vi "Steuerprogramm-Fr-13-01-17.vi"() -> ()   [LabVIEW 2010]
uses:
  Emil/Licor-Steuerung/HAGAR V/Licor-Steuerung/display/GUI_Cluster_sdv.ctl
  Emil/Licor-Steuerung/HAGAR V/Licor-Steuerung/display/GUI_Cluster_Parameter.ctl
  Emil/Licor-Steuerung/HAGAR V/Licor-Steuerung/control/Licor-Commands.ctl
  Emil/Licor-Steuerung/HAGAR V/Licor-Steuerung/control/Licor-Parameter.ctl
  Emil/Licor-Steuerung/LicorLI7000/conventions/Licor-Source.ctl
  Emil/Licor-Steuerung/HAGAR V/Licor-Steuerung/control/Licor-Pump.ctl
  Emil/Licor-Steuerung/HAGAR V/Licor-Steuerung/display/GUI_Cluster_Graph.ctl
  Emil/Licor-Steuerung/HAGAR V/Licor-Steuerung/control/Licor-Sequences.ctl
  <vilib>/rvi/interface/nirviMethod/nirviMethod.xnode
  C:/Users/HAGAR-IV/Desktop/Zeugs/markus/version feb 2012/FPGA Bitfiles/pertrasgcfpga2_FPGATarget_FPGA-Programm-01_A75D3647.lvbitx
  C:/Users/HAGAR-IV/Desktop/Zeugs/Johnny/pertrasgc fpga/FPGA-Programm-01-17.vi
  <vilib>/rvi/interface/common/niFpgaNodeNameForErrorReporting.ctl
  <vilib>/rvi/errors/niLvFpgaWhatHappensToTopLevelVI.ctl
  <vilib>/rvi/interface/nirviReadWriteControl/nirviReadWriteControl.xnode
  <vilib>/rvi/interface/nirviCloseFPGA/nirviCloseFPGA.xnode
  GVProbenvol.vi
  GVZeitenZyklen.vi
  GVECDs.vi
  GVZwangs.vi
  GVMethodenwechsel.vi
  GVTrapsMachs.vi
  GVHK1Hz.vi
  GVAIs.vi
  gvbooleschRT.vi
  GVMetavariablen.vi
  GVVentilposition.vi
  GVHorstSP.vi
  GVMWHorst.vi
  GVHeizenLH.vi
  <vilib>/Utility/error.llb/Error Cluster From Error Code.vi
  <vilib>/rvi/errors/niLvFpgaAdjustHostInterfaceError.vi
  GVaktuelleTDMS.vi
  Emil/Licor-Steuerung/HAGAR V/Licor-Steuerung/control/Emulate Licor output GV.vi
  GVChroms.vi
  GVZwangsMPV.vi
  <vilib>/FPGAPlugInAG/cRIO-9114/niLvFpga_Close_cRIO-9114.vi
  NiFpgaLv.dll
  Emil/Licor-Steuerung/HAGAR V/Licor-Steuerung/Licor-Steuerung.lvlib
  Emil/Licor-Steuerung/LicorLI7000/LicorLI7000.lvlib
panel:
  in  "Methode speichern":bool
  out "ZyklusNummernGesamt":i32[](array[numeric])
  in  "veränderte Methode benutzen":bool
  in  "Methode verändern":bool
  out "ZyklusNummern":i32[](array[numeric])
  out "Big Ben, Methodenzeit, Zykluszeit0, Zykluszeit1, Zykluszeit2A, Zykluszeit2B":i32[](array[numeric])
  in  "global stop RT":bool
  in  "Methode":i32(ring) items=["Bedingsmethode", "Startmethode", "Meßmodus", "Shut-up-Methode", "Test", "HAG2 1/2", "Startmethode", "HAG2 1/2 Aufwärmen", "LicorDruckProfil1", "LicorDruckProfil2", "LicorDruckProfil0", "LicorDruckProfil3"]
  in  "Registerkarte":T1(tab)
  out "SHOK?":bool[](array[boolean])
  out "schnelle Heizungen":string[](array[string])
  out "schnelle Heizungen":dbl[](array[numeric])
  out "HorstOK?":bool[](array[boolean])
  out "AIs3OK?":bool[](array[boolean])
  out "AIs1OK?":bool[](array[boolean])
  out "AIs1":dbl[](array[numeric])
  out "AIs1":string[](array[string])
  out "AIs2":string[](array[string])
  out "AIs3":string[](array[string])
  out "AIs2":dbl[](array[numeric])
  out "AIs3":dbl[](array[numeric])
  out "Metavariablen":string[](array[string])
  out "Metavariablen":dbl[](array[numeric])
  out "MWHorst":dbl[](array[numeric])
  out "HorstRegler":string[](array[string])
  out "AIs2OK?":bool[](array[boolean])
  out "Ventilposition":i32=1 min=1 max=6 step=1
  out "MVOK?":bool[](array[boolean])
  out "Housekeeping1":cluster{dbl[], dbl[]}(graph)
  in  "Zeitachse1":i32(ring)=1 items=["Zykluszeit [s] Mod0", "Zykluszeit [s] Mod1", "Zykluszeit [s] Mod2A", "Zykluszeit [s] Mod2B"]
  in  "dargestellte Größe 1":i32(ring)=1 items=["T1-Trap1 [°C]", "T1-Trap2 [°C]", "T1-StirlingKühlkopf [°C]", "T1-PreCol1 [°C]", "T1-PreCol2 [°C]", "T1-MainCol1a [°C]", "T1-MainCol1b [°C]", "T1-MainCol2a [°C]", "T1-MainCol2b [°C]", "T1-Bronkhorst1a [°C]", "T1-Bronkhorst1b [°C]", "T1-Bronkhorst2a [°C]", "T1-Bronkhorst2b [°C]", "T1-2Pos1B [°C]", "T1-Spare9", "T1-2Pos1A [°C]", "T1-Spare10", "T1-TurboPump [°C]", "T1-StirlingPlatine [°C]", "T1-Spare5", "T1-Spare6", "T1-Spare7", "T1-Spare8", "F1-MFM1", "F1-MFM0D [mL]", "P1-HeliumHP [bara]", "P1-HeliumLP [bara]", "P1-PumpVordruck [mbara]", "TurboSpeed", "I1-MS-AC [A]", "I1-Trap1 [A]", "I1-Trap2 [A]", "T2-ECD1a", "T2-ECD1b", "T2-ECD2a", "T2-ECD2b", "T2-Col1a", "T2-Col1b", "T2-Col2a", "T2-Col2b", "T2-Spare1", "T2-Spare2", "T2-Oven_a", "T2-Oven_b", "T2-Spare3", "T2-Spare4", "T2-Spare5", "F2-MFM0", "F2-MFM2A", "F2-MFM2B", "P2-N2O_HP", "P2-N2O_LP", "P2-CO2_HP", "P2-CO2_LP", "AI-Spare1", "FL-MFM1000mL", "AI-Spare3", "AI-Spare4", "StirlingAlarm", "StirlingEmerg.", "AI-Spare7", "AI-Spare8", "AI-Spare9", "FL-MFM30mL", "T0-DC/DC5", "I0-24V_M0", "I0-48V_M1", "I0-24V_M1", "I0-28V_M2", "T0-Spare3", "T0-Spare2", "T0-Spare4", "T0-DC/DC7", "I0-20V_Laptop", "I0-28V_M1", "I0-24V_M2", "I0-12V_Licor", "T0-Spare1", "T0-Drier", "T0-Spare5", "F0-MFM0A [L]", "TL-Licor_a", "P0-Span-HP", "P0-spare1", "P0-Stickstoff-LP", "P0-Helium-LP", "P0-Cal-HP", "P0-P9Tavco[bar]", "F0-MFM0B [L]", "TL-Licor_b", "P0-Span-LP", "P0-spare2", "P0-Stickstoff-HP", "P0-Helium-HP", "P0-Cal-LP", "F0-MFM3", "TemperaturTrap1[°C]", "TemperaturTrap2[°C]", "TemperaturPreMach1[°C]", "TemperaturPreMach2[°C]", "TemperaturMainMach1[°C]", "TemperaturMainMach2[°C]", "PrC0 [bara]", "PrC0-Licor [bara]", "PrC1-Säule1 [bara]", "PrC1-Säule2 [bara]", "MFC1-Sample [ml/min]", "PrC1-BackFlush1 [bara]", "PrC1-BackFlush2 [bara]", "MFC1-Reaktant [l/min]", "MFC2A[ml/min]", "MFC2B[ml/min]", "MFC2C[ul/min]", "PrC2A[bara]", "MFC2D[ml/min]", "MFC2E[ml/min]", "PrC2B[bara]"]
  out "Housekeeping2":cluster{dbl[], dbl[]}(graph)
  in  "Zeitachse2":i32(ring)=1 items=["Zykluszeit [s] Mod0", "Zykluszeit [s] Mod1", "Zykluszeit [s] Mod2A", "Zykluszeit [s] Mod2B"]
  in  "dargestellte Größe 2":i32(ring)=1 items=["T1-Trap1 [°C]", "T1-Trap2 [°C]", "T1-StirlingKühlkopf [°C]", "T1-PreCol1 [°C]", "T1-PreCol2 [°C]", "T1-MainCol1a [°C]", "T1-MainCol1b [°C]", "T1-MainCol2a [°C]", "T1-MainCol2b [°C]", "T1-Bronkhorst1a [°C]", "T1-Bronkhorst1b [°C]", "T1-Bronkhorst2a [°C]", "T1-Bronkhorst2b [°C]", "T1-2Pos1B [°C]", "T1-Spare9", "T1-2Pos1A [°C]", "T1-Spare10", "T1-TurboPump [°C]", "T1-StirlingPlatine [°C]", "T1-Spare5", "T1-Spare6", "T1-Spare7", "T1-Spare8", "F1-MFM1", "F1-MFM0D [mL]", "P1-HeliumHP [bara]", "P1-HeliumLP [bara]", "P1-PumpVordruck [mbara]", "TurboSpeed", "I1-MS-AC [A]", "I1-Trap1 [A]", "I1-Trap2 [A]", "T2-ECD1a", "T2-ECD1b", "T2-ECD2a", "T2-ECD2b", "T2-Col1a", "T2-Col1b", "T2-Col2a", "T2-Col2b", "T2-Spare1", "T2-Spare2", "T2-Oven_a", "T2-Oven_b", "T2-Spare3", "T2-Spare4", "T2-Spare5", "F2-MFM0", "F2-MFM2A", "F2-MFM2B", "P2-N2O_HP", "P2-N2O_LP", "P2-CO2_HP", "P2-CO2_LP", "AI-Spare1", "FL-MFM1000mL", "AI-Spare3", "AI-Spare4", "StirlingAlarm", "StirlingEmerg.", "AI-Spare7", "AI-Spare8", "AI-Spare9", "FL-MFM30mL", "T0-DC/DC5", "I0-24V_M0", "I0-48V_M1", "I0-24V_M1", "I0-28V_M2", "T0-Spare3", "T0-Spare2", "T0-Spare4", "T0-DC/DC7", "I0-20V_Laptop", "I0-28V_M1", "I0-24V_M2", "I0-12V_Licor", "T0-Spare1", "T0-Drier", "T0-Spare5", "F0-MFM0A [L]", "TL-Licor_a", "P0-Span-HP", "P0-spare1", "P0-Stickstoff-LP", "P0-Helium-LP", "P0-Cal-HP", "P0-P9Tavco[bar]", "F0-MFM0B [L]", "TL-Licor_b", "P0-Span-LP", "P0-spare2", "P0-Stickstoff-HP", "P0-Helium-HP", "P0-Cal-LP", "F0-MFM3", "TemperaturTrap1[°C]", "TemperaturTrap2[°C]", "TemperaturPreMach1[°C]", "TemperaturPreMach2[°C]", "TemperaturMainMach1[°C]", "TemperaturMainMach2[°C]", "PrC0 [bara]", "PrC0-Licor [bara]", "PrC1-Säule1 [bara]", "PrC1-Säule2 [bara]", "MFC1-Sample [ml/min]", "PrC1-BackFlush1 [bara]", "PrC1-BackFlush2 [bara]", "MFC1-Reaktant [l/min]", "MFC2A[ml/min]", "MFC2B[ml/min]", "MFC2C[ul/min]", "PrC2A[bara]", "MFC2D[ml/min]", "MFC2E[ml/min]", "PrC2B[bara]"]
  out "Detektor 2":cluster{dbl[], dbl[]}[](graph)
  in  "Detektor":i32(ring) items=["ECD1", "ECD2"]
  in  "HK1YMin":dbl
  in  "HK1YMax":dbl=100.0
  in  "HK2YMin":dbl
  in  "HK2YMax":dbl=100.0
  in  "DetYMin":dbl
  in  "DetYMax":dbl=100.0
  out "schnelleAnzeige":cluster{dbl[], dbl[]}(graph)
  in  "TafelWischen!":bool
  in  "dargestellte Größe 3":i32(ring)=1 items=["TemperaturTrap1[°C]", "TemperaturTrap2[°C]", "TemperaturPreMach1[°C]", "TemperaturPreMach2[°C]", "TemperaturMainMach1[°C]", "TemperaturMainMach2[°C]", "PrC0 [bara]", "PrC0-Licor [bara]", "PrC1-Säule1 [bara]", "PrC1-Säule2 [bara]", "MFC1-Sample [ml/min]", "PrC1-BackFlush1 [bara]", "PrC1-BackFlush2 [bara]", "MFC1-Reaktant [l/min]", "MFC2A[ml/min]", "MFC2B[ml/min]", "MFC2C[ul/min]", "PrC2A[bara]", "MFC2D[ml/min]", "MFC2E[ml/min]", "PrC2B[bara]"]
  in  "An/Aus":bool
  in  "Registerkarte 2":T2(tab)
  in  "GUI_Cluster_Graph":T3={"time (global)"=0.0, "command queue"=[], "Rohdaten"=[], "Graph"={"X"=[], "Y"=[]}, "Manuelle Steuerung"={"Sequenz"=enum."test", "Manuelle Steuerung An/Aus"=FALSE}, "Sequenz out"={"sequence"=enum."WAIT", "Zeitpunkt next"=0.0, "delta t"=0.0}} caption="Cluster" {"Sequenz out"."Zeitpunkt next" format="%<%H:%M:%S%3u>T"; "time (global)" format="%<%H:%M:%S%3u\n%m/%d/%y>T"}
  in  "GUI_Cluster_Parameter":T5={"warmup (sequence)"=[{"time"=60, "Enum"=enum."wait"}], "calibrate S (sequence)"=[{"time"=60, "Enum"=enum."wait"}, {"time"=2, "Enum"=enum."getCalibrationParameter"}, {"time"=8, "Enum"=enum."calibration-S-CO2"}, {"time"=2, "Enum"=enum."getCalibrationParameter"}], "calibrate Z (sequence)"=[{"time"=60, "Enum"=enum."wait"}, {"time"=2, "Enum"=enum."getCalibrationParameter"}, {"time"=8, "Enum"=enum."calibration-Z-H2O"}, {"time"=2, "Enum"=enum."getCalibrationParameter"}, {"time"=8, "Enum"=enum."calibration-Z-CO2"}, {"time"=2, "Enum"=enum."getCalibrationParameter"}], "initialize (sequence)"=[{"time"=30, "Enum"=enum."wait"}, {"time"=2, "Enum"=enum."setPumpSlow"}, {"time"=2, "Enum"=enum."setPumpMedium"}, {"time"=2, "Enum"=enum."setPumpFast"}, {"time"=10, "Enum"=enum."initialize"}, {"time"=4, "Enum"=enum."getCalibrationParameter"}, {"time"=2, "Enum"=enum."resetH2O"}, {"time"=4, "Enum"=enum."resetCO2"}, {"time"=4, "Enum"=enum."getCalibrationParameter"}, {"time"=2, "Enum"=enum."setZeroParameter"}, {"time"=4, "Enum"=enum."getCalibrationParameter"}, {"time"=2, "Enum"=enum."setReference"}, {"time"=4, "Enum"=enum."getLicorTime"}, {"time"=5, "Enum"=enum."getInfo"}], "Licor-parameter"={"CO2 ref"=402.3, "CO2 span"=392.3, "H2O ref"=0.0, "H2O span"=0.0, "Zi"=1.2, "Zt"=6.494e-05, "Zm"=0.0, "S"=1.34, "Temp [C]"=45.0, "Pressure [hPa]"=1013.0, "Licor-Sources"=["CO2A W", "CO2B W", "H2OA W", "H2OB W", "T C", "T V", "P kPa", "P V", "RH %", "CO2A um/m", "CO2B um/m", "H2OA mm/m", "H2OB mm/m"], "Licor-Pump"="Off", "Zeitstempel"=timestamp(0 s since 1904-01-01)}} {"Licor-parameter"."Pressure [hPa]" format="%_5g"; "Licor-parameter"."Temp [C]" format="%.2f"; "Licor-parameter"."CO2 ref" format="%.2f"; "Licor-parameter"."CO2 span" format="%.2g"; "Licor-parameter"."H2O ref" format="%.2g"; "Licor-parameter"."H2O span" format="%.2g"; "Licor-parameter"."Zt" format="%#_4g"}
  in  "GUI_Cluster_sdv":T10={"Graph_sdv"={"X"=[], "Y"=[]}, "Breite"=20, "Berechnen"=FALSE, "residue"=0.0} {"residue" format="%_6g"}
  in  "VISA resource name":refnum<visa-resource-name>="ASRL1::INSTR" caption="VISA-Ressourcenname"
  in  "ServosWarmHigh (us)KaltHigh(us)":T11={"Servo1WarmHigh(us)"=1000, "Servo1KaltHigh(us)"=1000, "Servo2WarmHigh(us)"=2030, "Servo2KaltHigh(us)"=2030}
  out "TDMSwriteECD":errorcluster
  out "AIsFIFOread":errorcluster
  out "MWTrapsMachs":errorcluster
  out "TDMSwriteHK":errorcluster
  out "TDMScloseHK":errorcluster
  out "TDMSopenHK":errorcluster
  out "TDMScloseECD2":errorcluster
  out "TDMSopenECD2":errorcluster
  out "TDMScloseECD1":errorcluster
  out "TDMSopenECD1":errorcluster
  out "FIFOwriteRS485":errorcluster
  out "SerielleKomm.":errorcluster
  out "LH":errorcluster
  out "Zyklus":errorcluster
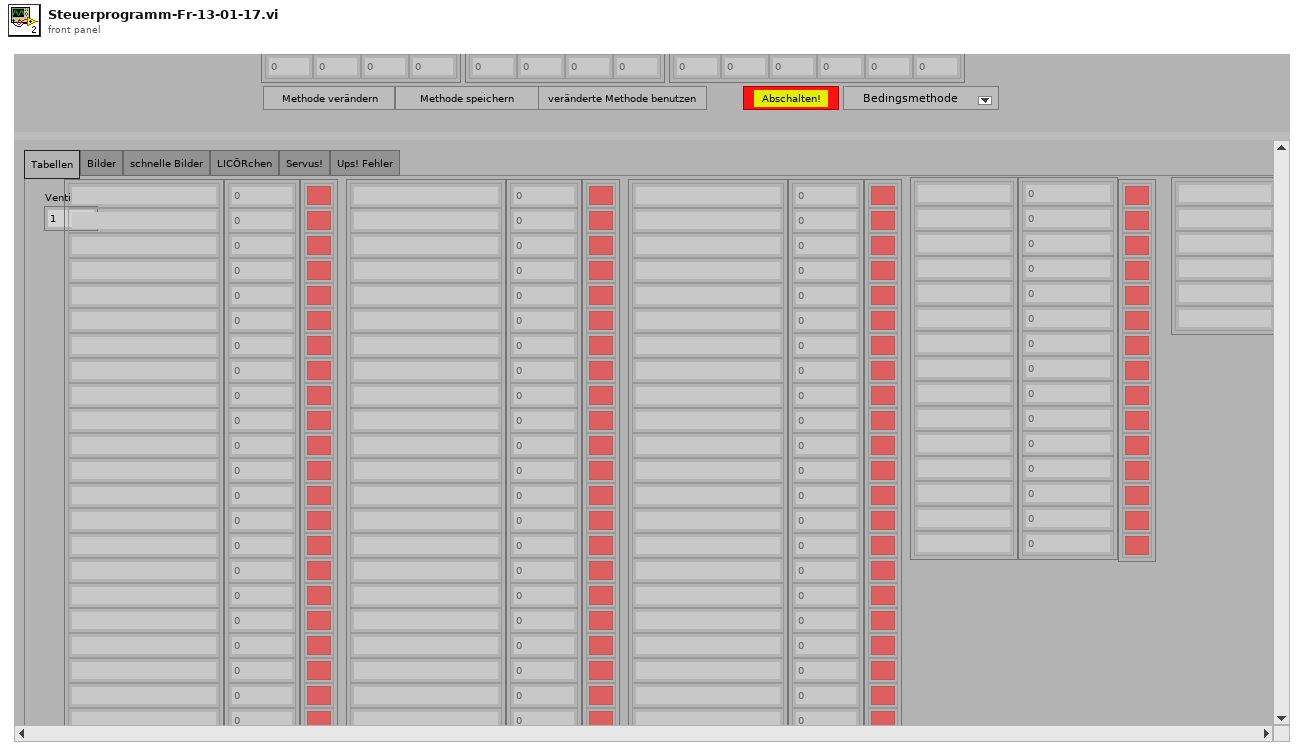
[diagram p1: front panel]
types:
  T1 = enum32{"Tabellen", "Bilder", "schnelle Bilder", "LICÖRchen", "Servus!", "Ups! Fehler"}
  T2 = enum32{"Graph", "Parameter / Sequenzen", "sdv", "debug"}
  T3 = typedef "Licor-Steuerung.lvlib/GUI_Cluster_Graph.ctl" = cluster{"time (global)":dbl, "command queue":cluster{"Zeit [s]":i32, "Befehl":string}[], "Rohdaten":string[], "Graph":cluster{"X":dbl[], "Y":dbl[]}, "Manuelle Steuerung":cluster{"Sequenz":T4, "Manuelle Steuerung An/Aus":bool}, "Sequenz out":cluster{"sequence":T4, "Zeitpunkt next":dbl, "delta t":dbl}}
  T4 = typedef "Licor-Steuerung.lvlib/Licor-Sequences.ctl" = enum16{"test", "WAIT", "warmup", "initialize", "calibrate Z", "calibrate S"}
  T5 = typedef "Licor-Steuerung.lvlib/GUI_Cluster_Parameter.ctl" = cluster{"warmup (sequence)":cluster{"time":i32, "Enum":T6}[], "calibrate S (sequence)":cluster{"time":i32, "Enum":T6}[], "calibrate Z (sequence)":cluster{"time":i32, "Enum":T6}[], "initialize (sequence)":cluster{"time":i32, "Enum":T6}[], "Licor-parameter":T7}
  T6 = typedef "Licor-Steuerung.lvlib/Licor-Commands.ctl" = enum16{"wait", "initialize", "resetCO2", "resetH2O", "getReference", "setReference", "calibration-Z-CO2", "calibration-Z-H2O", "calibration-S-CO2", "calibration-S-H2O", "getCalibrationParameter", "setZeroParameter", "setLicorTime", "getLicorTime", "setPumpFlowrate", "setPumpSlow", "setPumpMedium", "setPumpFast", "getInfo"}
  T7 = typedef "Licor-Steuerung.lvlib/Licor-Parameter.ctl" = cluster{"CO2 ref":dbl, "CO2 span":dbl, "H2O ref":dbl, "H2O span":dbl, "Zi":dbl, "Zt":dbl, "Zm":dbl, "S":dbl, "Temp [C]":dbl, "Pressure [hPa]":dbl, "Licor-Sources":T8[], "Licor-Pump":T9, "Zeitstempel":timestamp}
  T8 = typedef "LicorLI7000.lvlib/Licor-Source.ctl" = string
  T9 = typedef "Licor-Steuerung.lvlib/Licor-Pump.ctl" = string
  T10 = typedef "Licor-Steuerung.lvlib/GUI_Cluster_sdv.ctl" = cluster{"Graph_sdv":cluster{"X":dbl[], "Y":dbl[]}, "Breite":i32, "Berechnen":bool, "residue":dbl}
  T11 = cluster{"Servo1WarmHigh(us)":u32, "Servo1KaltHigh(us)":u32, "Servo2WarmHigh(us)":u32, "Servo2KaltHigh(us)":u32}
  T12 = cluster{"DIOsMod0Nr":i32[], "DIOsMod1Nr":i32[], "DIOsMod2ANr":i32[], "DIOsMod2BNr":i32[], "AIsLH":i32[], "AnzahlRegler/Modul":i32[], "Regler für den Probenfluß":i32, "SPvorgebenMod0":string[], "SPvorgebenMod1":string[], "SPvorgebenMod2A":string[], "SPvorgebenMod2B":string[], "MWAntwortMod0":string[], "MWAntwortMod1":string[], "MWAntwortMod2A":string[], "MWAntwortMod2B":string[], "FaktorMod0":dbl[], "FaktorMod1":dbl[], "FaktorMod2A":dbl[], "FaktorMod2B":dbl[], "MWabfragenMod0":string[], "MWabfragenMod1":string[], "MWabfragenMod2A":string[], "MWabfragenMod2B":string[], "Modul1/AI koeff":dbl[][], "Modul2/AI koeff":dbl[][], "Modul3/AI koeff":dbl[][], "Traps/MachsKoeff":dbl[][], "Modul1/AIsNamen":string[], "Modul2/AIsNamen":string[], "Modul3/AIsNamen":string[], "DIOsMod0Name":string[], "DIOsMod1Name":string[], "DIOsMod2AName":string[], "DIOsMod2BName":string[], "ReglerNameMod0":string[], "ReglerNameMod1":string[], "ReglerNameMod2A":string[], "ReglerNameMod2B":string[], "Startmethode":i32, "Dateiordner Housekeeping":path, "Dateiname Housekeeping":string, "DateiordnerECD1":path, "DateinameECD1":string, "DateiordnerECD2":path, "DateinameECD2":string, "LangsameHeizungen":string[], "ModuleLH":i32[], "Metavariablen":string[], "Modul1/AI sicherer Bereich":dbl[][], "Modul2/AI sicherer Bereich":dbl[][], "Modul3/AI sicherer Bereich":dbl[][], "Traps/Machs sicherer Bereich":dbl[][], "ReglerMod0 sicherer Bereich":dbl[][], "ReglerMod1 sicherer Bereich":dbl[][], "ReglerMod2A sicherer Bereich":dbl[][], "ReglerMod2B sicherer Bereich":dbl[][], "Metavariablen grüner Bereich":dbl[][]}
  T13 = cluster{"Zykluslängen [s]":dbl[], "ZeitpktDIOsMod0":dbl[], "ZeitpktDIOsMod1":dbl[], "ZeitpktDIOsMod2A":dbl[], "ZeitpktDIOsMod2B":dbl[], "DIOsSPMod0":bool[][], "DIOsSPMod1":bool[][], "DIOsSPMod2A":bool[][], "DIOsSPMod2B":bool[][], "Mod0HorstZeitpkt":dbl[], "Mod1HorstZeitpkt":dbl[], "Mod2AHorstZeitpkt":dbl[], "Mod2BHorstZeitpkt":dbl[], "HorstSPMod0":dbl[][], "HorstSPMod1":dbl[][], "HorstSPMod2A":dbl[][], "HorstSPMod2B":dbl[][], "LHSetpoints":dbl[], "LHHeizen?":bool[], "ZPktFPGABoolesch":dbl[], "FPGABoolesch":bool[][], "ZeitpktFPGAPID":dbl[], "FPGAPID":cluster{"proportional gain (Kc)":fxp<+/-,16,8>, "integral gain (Kc*Ts/Ti)":fxp<+/-,16,8>, "derivative gain (Kc*Td/Ts)":fxp<+/-,16,8>}[][], "ZeitpktFPGAFixp":dbl[], "SHSetpoints":dbl[][], "t_PreMach1":dbl[], "T_PreMach1":dbl[], "t_PreMach2":dbl[], "T_PreMach2":dbl[], "PIDs für \"träge\" Heizungen":cluster{"proportional gain (Kc)":dbl, "integral time (Ti, min)":dbl, "derivative time (Td, min)":dbl}[], "Zwangsbedingungen":dbl[][], "Dateien fürs MS schicken?":bool, "ZeitpunkteMPV":dbl[], "SPMPV":i32[], "ZeitpktMS-1":dbl, "ZeitpktMS-2":dbl, "Int.Start1":dbl, "Int.Stop1":dbl, "Int.Start2":dbl, "Int.Stop2":dbl, "Methodenname":string, "t_MainMach1":dbl[], "T_MainMach1":dbl[], "t_MainMach2":dbl[], "T_MainMach2":dbl[]}[]
  T14 = enum16{"open", "replace", "create", "open or create", "replace or create", "replace or create with confirmation"}
  T15 = typedef "niFpgaNodeNameForErrorReporting.ctl" = enum16{"Open FPGA VI Reference", "Read/Write Control", "Invoke Method: Abort", "Invoke Method: Acknowledge IRQ", "Invoke Method: Download", "Invoke Method: FIFO.Configure", "Invoke Method: FIFO.Read", "Invoke Method: FIFO.Start", "Invoke Method: FIFO.Stop", "Invoke Method: FIFO.Write", "Invoke Method: Reset", "Invoke Method: Run", "Invoke Method: Wait on IRQ", "Close FPGA VI Reference"}
  T16 = typedef "niLvFpgaWhatHappensToTopLevelVI.ctl" = enum16{"top level VI scripted behind XNode", "top level VI inlined behind XNode"}
  T17 = cluster{"Zyklus1":i32, "Zeitachse1":i32, "dargestellte Größe 1":i32, "Zyklus2":i32, "Zeitachse2":i32, "dargestellte Größe 2":i32}
  T18 = cluster{"Modul1/AI sicherer Bereich":dbl[][], "Modul2/AI sicherer Bereich":dbl[][], "Modul3/AI sicherer Bereich":dbl[][], "Traps/Machs sicherer Bereich":dbl[][], dbl[][], "Metavariablen grüner Bereich":dbl[][]}
  T19 = cluster{"DIOsMod0Name":string[], "DIOsMod1Name":string[], "DIOsMod2AName":string[], "DIOsMod2BName":string[], "ReglerNameMod0":string[], "ReglerNameMod1":string[], "ReglerNameMod2A":string[], "ReglerNameMod2B":string[], "LangsameHeizungen":string[]}
  T20 = cluster{"Zykluslängen [s]":dbl[], "ZeitpktDIOsMod0":dbl[], "ZeitpktDIOsMod1":dbl[], "ZeitpktDIOsMod2A":dbl[], "ZeitpktDIOsMod2B":dbl[], "DIOsSPMod0":bool[][], "DIOsSPMod1":bool[][], "DIOsSPMod2A":bool[][], "DIOsSPMod2B":bool[][], "Mod0HorstZeitpkt":dbl[], "Mod1HorstZeitpkt":dbl[], "Mod2AHorstZeitpkt":dbl[], "Mod2BHorstZeitpkt":dbl[], "HorstSPMod0":dbl[][], "HorstSPMod1":dbl[][], "HorstSPMod2A":dbl[][], "HorstSPMod2B":dbl[][], "LHSetpoints":dbl[], "LHHeizen?":bool[], "ZPktFPGABoolesch":dbl[], "FPGABoolesch":bool[][], "ZeitpktFPGAPID":dbl[], "FPGAPID":cluster{"proportional gain (Kc)":fxp<+/-,16,8>, "integral gain (Kc*Ts/Ti)":fxp<+/-,16,8>, "derivative gain (Kc*Td/Ts)":fxp<+/-,16,8>}[][], "ZeitpktFPGAFixp":dbl[], "SHSetpoints":dbl[][], "t_PreMach1":dbl[], "T_PreMach1":dbl[], "t_PreMach2":dbl[], "T_PreMach2":dbl[], "PIDs für \"träge\" Heizungen":cluster{"proportional gain (Kc)":dbl, "integral time (Ti, min)":dbl, "derivative time (Td, min)":dbl}[], "Zwangsbedingungen":dbl[][], "Dateien fürs MS schicken?":bool, "ZeitpunkteMPV":dbl[], "SPMPV":i32[], "ZeitpktMS-1":dbl, "ZeitpktMS-2":dbl, "Int.Start1":dbl, "Int.Stop1":dbl, "Int.Start2":dbl, "Int.Stop2":dbl, "Methodenname":string, "t_MainMach1":dbl[], "T_MainMach1":dbl[], "t_MainMach2":dbl[], "T_MainMach2":dbl[]}
  T21 = cluster{"created path":path, "created path":path, "created path":path, "Dateiname Housekeeping":string, "DateinameECD1":string, "DateinameECD2":string, "tdms0":refnum<k34>, "tdms1":refnum<k34>, "tdms0":refnum<k34>, "tdms1":refnum<k34>, "tdms0":refnum<k34>, "tdms1":refnum<k34>}
  T22 = cluster{"proportional gain (Kc)":fxp<+/-,16,8>, "integral gain (Kc*Ts/Ti)":fxp<+/-,16,8>, "derivative gain (Kc*Td/Ts)":fxp<+/-,16,8>}[][]
  T23 = cluster{"proportional gain (Kc)":dbl, "integral time (Ti, min)":dbl, "derivative time (Td, min)":dbl}[]
  T24 = cluster{cluster{"ZeitpktDIOsMod2B":dbl[]}[], cluster{"DIOsSPMod2B":bool[][]}[], cluster{"Mod2BHorstZeitpkt":dbl[]}[], cluster{"HorstSPMod2B":dbl[][]}[], "LHHeizen?":bool[], "ZPktFPGABoolesch":dbl[], "FPGABoolesch":bool[][], "ZeitpktFPGAPID":dbl[], "FPGAPID":cluster{"proportional gain (Kc)":fxp<+/-,16,8>, "integral gain (Kc*Ts/Ti)":fxp<+/-,16,8>, "derivative gain (Kc*Td/Ts)":fxp<+/-,16,8>}[][], "ZeitpktFPGAFixp":dbl[], "SHSetpoints":dbl[][], "t_PreMach1":dbl[], "T_PreMach1":dbl[], "t_PreMach2":dbl[], "T_PreMach2":dbl[], "ZeitpunkteMPV":dbl[], "SPMPV":i32[], "t_MainMach1":dbl[], "T_MainMach1":dbl[], "t_MainMach2":dbl[], "T_MainMach2":dbl[]}
  T25 = cluster{"Zykluslängen [s]":dbl[], "ZeitpktDIOsMod0":dbl[], "ZeitpktDIOsMod1":dbl[], "ZeitpktDIOsMod2A":dbl[], "ZeitpktDIOsMod2B":dbl[], "DIOsSPMod0":bool[][], "DIOsSPMod1":bool[][], "DIOsSPMod2A":bool[][], "DIOsSPMod2B":bool[][], "Mod0HorstZeitpkt":dbl[], "Mod1HorstZeitpkt":dbl[], "Mod2AHorstZeitpkt":dbl[], "Mod2BHorstZeitpkt":dbl[], "HorstSPMod0":dbl[][], "HorstSPMod1":dbl[][], "HorstSPMod2A":dbl[][], "HorstSPMod2B":dbl[][], "LangsameHeizungenSP":dbl[], "LHHeizen?":bool[], "ZPktFPGABoolesch":dbl[], "FPGABoolesch":bool[][], "ZeitpktFPGAPID":dbl[], "FPGAPID":cluster{"proportional gain (Kc)":fxp<+/-,16,8>, "integral gain (Kc*Ts/Ti)":fxp<+/-,16,8>, "derivative gain (Kc*Td/Ts)":fxp<+/-,16,8>}[][], "ZeitpktFPGAFixp":dbl[], "FPGAFixp":dbl[][], "t_PreMach1":dbl[], "T_PreMach1":dbl[], "t_PreMach2":dbl[], "T_PreMach2":dbl[], "PIDs für \"träge\" Heizungen":cluster{"proportional gain (Kc)":dbl, "integral time (Ti, min)":dbl, "derivative time (Td, min)":dbl}[], "Zwangsbedingungen":dbl[][], "MS-Daten?":bool, "ZeitpunkteMPV":dbl[], "SetpointMPV":i32[], "ZeitpktMS-1":dbl, "ZeitpktMS-2":dbl, "Int.Start1":dbl, "Int.Stop1":dbl, "Int.Start2":dbl, "Int.Stop2":dbl, "Methodenname":string, "t_MainMach1":dbl[], "T_MainMach1":dbl[], "t_MainMach2":dbl[], "T_MainMach2":dbl[]}
  T26 = cluster{"ZyklusNummern":i32[], "ZeilennummernDIOs":i32[], "ZwangsDIO?":cluster{bool[]}[], "ZeilennummernHorst":i32[], "ZwangsHorst?":cluster{bool[]}[], "ZeileFPGABoolesch":i32, "ZwangsFPGABoolesch?":bool[], "ZeileFPGAPID":i32, "ZeileFPGAFixp":i32, "ZeilePreMach1":i32, "ZeilePreMach2":i32, "ZeilennummerMPV":i32, "ZeileMainMach1":i32, "ZeileMainMach2":i32, "ZwangsMPV?":bool}
  T27 = cluster{"ZyklusNummern":i32[], i32[], "ZwangsDIO?":cluster{bool[]}[], i32[], "ZwangsHorst?":cluster{bool[]}[], i32, "ZwangsFPGABoolesch?":bool[], i32, i32, "ZeileMach":i32, "ZeileMach":i32, i32, "ZeileMach":i32, "ZeileMach":i32, "ZwangsMPV?":bool}
  T28 = cluster{string[], string[], string[], dbl[], dbl[], dbl[]}
  T29 = cluster{"Befehle1":string[], "Befehle2":string[], "Befehle3":string[]}
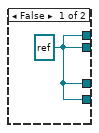
[diagram p2: hidden frame]
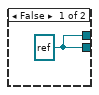
[diagram p3: hidden frame]
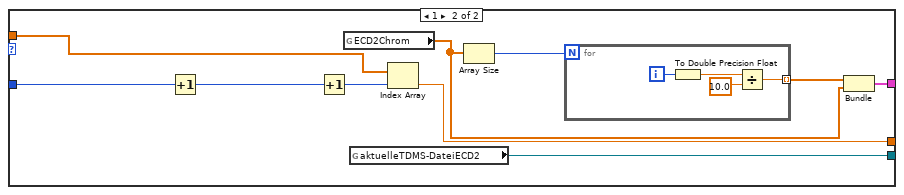
[diagram p12: hidden frame]
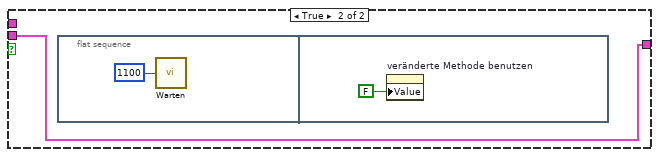
[diagram p13: hidden frame]
diagram:
  n1 = Open/Create/Replace File(file path (use dialog)=path "c:/einstellungen.perx" ("Datei (Dialog verwenden)"), operation (0:open)=T14."open" ("Operation (0:Öffnen)")) -> (refnum out=w13:refnum<file>)  [unwired: 4 in, 2 out]
  n2 = Open/Create/Replace File(file path (use dialog)=path "c:/methoden.per" ("Datei (Dialog verwenden)"), operation (0:open)=T14."open" ("Operation (0:Öffnen)")) -> (refnum out=w8:refnum<file>)  [unwired: 4 in, 2 out]
  n3 = Read from Binary File(5:T12 {"DIOsMod0Nr"=[], "DIOsMod1Nr"=[], "DIOsMod2ANr"=[], "DIOsMod2BNr"=[], "AIsLH"=[], "AnzahlRegler/Modul"=[], "Regler für den Probenfluß"=0, "SPvorgebenMod0"=[], "SPvorgebenMod1"=[], "SPvorgebenMod2A"=[], "SPvorgebenMod2B"=[], "MWAntwortMod0"=[], "MWAntwortMod1"=[], "MWAntwortMod2A"=[], "MWAntwortMod2B"=[], "FaktorMod0"=[], "FaktorMod1"=[], "FaktorMod2A"=[], "FaktorMod2B"=[], "MWabfragenMod0"=[], "MWabfragenMod1"=[], "MWabfragenMod2A"=[], "MWabfragenMod2B"=[], "Modul1/AI koeff"=[], "Modul2/AI koeff"=[], "Modul3/AI koeff"=[], "Traps/MachsKoeff"=[], "Modul1/AIsNamen"=[], "Modul2/AIsNamen"=[], "Modul3/AIsNamen"=[], "DIOsMod0Name"=[], "DIOsMod1Name"=[], "DIOsMod2AName"=[], "DIOsMod2BName"=[], "ReglerNameMod0"=[], "ReglerNameMod1"=[], "ReglerNameMod2A"=[], "ReglerNameMod2B"=[], "Startmethode"=0, "Dateiordner Housekeeping"=path "", "Dateiname Housekeeping"="", "DateiordnerECD1"=path "", "DateinameECD1"="", "DateiordnerECD2"=path "", "DateinameECD2"="", "LangsameHeizungen"=[], "ModuleLH"=[], "Metavariablen"=[], "Modul1/AI sicherer Bereich"=[], "Modul2/AI sicherer Bereich"=[], "Modul3/AI sicherer Bereich"=[], "Traps/Machs sicherer Bereich"=[], "ReglerMod0 sicherer Bereich"=[], "ReglerMod1 sicherer Bereich"=[], "ReglerMod2A sicherer Bereich"=[], "ReglerMod2B sicherer Bereich"=[], "Metavariablen grüner Bereich"=[]} ("output cluster"), 11:w13) -> (2:w11:T12, 3:w12:refnum<file>)  [unwired: 4 in, 2 out]
  n4 = Read from Binary File(5:T13 [], 11:w8) -> (2:w6:T13, 3:w7:refnum<file>)  [unwired: 4 in, 2 out]
  n5 = Close File(refnum=w12) -> ()  [unwired: 1 in, 2 out]
  n6 = Close File(refnum=w7) -> ()  [unwired: 1 in, 2 out]
  n7 = flat-sequence {
    tunnel: [w54] -> w41
    tunnel: [w111] -> w40
    tunnel: [w58] -> w38
    tunnel: [w245] -> w37
    tunnel: [w247] -> w36
    tunnel: [w239] -> w35
    tunnel: [w246] -> w34
    tunnel: [w169] -> w33
    tunnel: [w238] -> w32
    tunnel: [w237] -> w31
    tunnel: [w231] -> w30
    tunnel: [w172] -> w29
    tunnel: [w146] -> w28
    tunnel: [w244] -> w27
    tunnel: [w236] -> w26
    tunnel: [w235] -> w25
    tunnel: [w227] -> w24
    tunnel: [w226] -> w23
    tunnel: [w225] -> w22
    tunnel: [w224] -> w21
    tunnel: [w223] -> w20
    tunnel: [w222] -> w19
    tunnel: [w219] -> w18
    tunnel: [w201] -> w17
    tunnel: w11 -> [w87]
    tunnel: [w200] -> w16
    tunnel: w6 -> [w112]
    tunnel: [w111] -> w5
    tunnel: [w87] -> w3
    tunnel: [w49] -> w1
    tunnel: w41 -> [w444]
    tunnel: w40 -> [w517]
    tunnel: [w444] -> w39
    tunnel: w38 -> [_]
    tunnel: w37 -> [w475]
    tunnel: w36 -> [w474]
    tunnel: w35 -> [w476]
    tunnel: w34 -> [w473]
    tunnel: w33 -> [w448]
    tunnel: w32 -> [w443]
    tunnel: w31 -> [w440]
    tunnel: w30 -> [w437]
    tunnel: w29 -> [w438]
    tunnel: w28 -> [w441]
    tunnel: w27 -> [w515]
    tunnel: w26 -> [w446]
    tunnel: w25 -> [w516]
    tunnel: w24 -> [w419]
    tunnel: w23 -> [w418]
    tunnel: w22 -> [w417]
    tunnel: w21 -> [w513]
    tunnel: w20 -> [w512]
    tunnel: w19 -> [w511]
    tunnel: w18 -> [w465]
    tunnel: w17 -> [w447]
    tunnel: w16 -> [w436]
    tunnel: w6 -> [w435]
    tunnel: w5 -> [w433]
    tunnel: w3 -> [_]
    tunnel: w1 -> [w412]
    tunnel: w39 -> [w1335]
    frame #0 {
      w113 = TRUE
      w128 = 0.0 ("Probenvol.1")
      w135 = dbl[] [-1.0] ("ECD1MW")
      w136 = FALSE ("ECD1Empfangen?")
      w127 = string[] ["TemperaturTrap1[°C]", "TemperaturTrap2[°C]", "TemperaturPreMach1[°C]", "TemperaturPreMach2[°C]", "TemperaturMainMach1[°C]", "TemperaturMainMach2[°C]"]
      w242 = string[] ["Big Ben [s]", "Methodenzeit [s]", "Zykluszeit [s] Mod0", "Zykluszeit [s] Mod1", "Zykluszeit [s] Mod2A", "Zykluszeit [s] Mod2B"]
      w232 = FALSE ("Undefinierte Werte möglich")
      w233 = FALSE ("global stop RT")
      n8 = for {
        tunnel: [w407] -> w240 mode=indexing
        tunnel: w112 -> [w408] mode=indexing
        n9 = Unbundle(w408) -> ("Methodenname"=w407:string)  [unwired: 44 out]
      }
      n10 = call "FPGA-Start-01-17.vi"() -> ("error out"=w58:errorcluster, "FPGA VI Reference Out"=w57:refnum<k20>)  [unwired: 2 in]
      n11 = Unbundle(w87) -> ("DIOsMod0Nr"=w156:i32[], "DIOsMod1Nr"=w155:i32[], "DIOsMod2ANr"=w154:i32[], "DIOsMod2BNr"=w153:i32[], "AIsLH"=w143:i32[], "AnzahlRegler/Modul"=w146:i32[], "Regler für den Probenfluß"=w200:i32, "SPvorgebenMod0"=w199:string[], "SPvorgebenMod1"=w198:string[], "SPvorgebenMod2A"=w197:string[], "SPvorgebenMod2B"=w196:string[], "MWAntwortMod0"=w195:string[], "MWAntwortMod1"=w194:string[], "MWAntwortMod2A"=w193:string[], "MWAntwortMod2B"=w192:string[], "FaktorMod0"=w191:dbl[], "FaktorMod1"=w190:dbl[], "FaktorMod2A"=w189:dbl[], "FaktorMod2B"=w188:dbl[], "MWabfragenMod0"=w187:string[], "MWabfragenMod1"=w186:string[], "MWabfragenMod2A"=w185:string[], "MWabfragenMod2B"=w184:string[], "Modul1/AI koeff"=w183:dbl[][], "Modul2/AI koeff"=w182:dbl[][], "Modul3/AI koeff"=w181:dbl[][], "Traps/MachsKoeff"=w180:dbl[][], "Modul1/AIsNamen"=w179:string[], "Modul2/AIsNamen"=w178:string[], "Modul3/AIsNamen"=w177:string[], "DIOsMod0Name"=w85:string[], "DIOsMod1Name"=w86:string[], "DIOsMod2AName"=w84:string[], "DIOsMod2BName"=w83:string[], "ReglerNameMod0"=w102:string[], "ReglerNameMod1"=w101:string[], "ReglerNameMod2A"=w100:string[], "ReglerNameMod2B"=w99:string[], "Startmethode"=w111:i32, "Dateiordner Housekeeping"=w82:path, "Dateiname Housekeeping"=w176:string, "DateiordnerECD1"=w96:path, "DateinameECD1"=w175:string, "DateiordnerECD2"=w95:path, "DateinameECD2"=w174:string, "LangsameHeizungen"=w173:string[], "ModuleLH"=w168:i32[], "Metavariablen"=w106:string[], "Modul1/AI sicherer Bereich"=w53:dbl[][], "Modul2/AI sicherer Bereich"=w52:dbl[][], "Modul3/AI sicherer Bereich"=w51:dbl[][], "Traps/Machs sicherer Bereich"=w50:dbl[][], "ReglerMod0 sicherer Bereich"=w48:dbl[][], "ReglerMod1 sicherer Bereich"=w47:dbl[][], "ReglerMod2A sicherer Bereich"=w46:dbl[][], "ReglerMod2B sicherer Bereich"=w45:dbl[][], "Metavariablen grüner Bereich"=w43:dbl[][])
      "Metavariablen" <- w106
      n12 = Initialize Array(0, 4 ("Dimension")) -> (w129:i32[])
      n13 = Initialize Array(0.0 ("Element"), 6 ("Dimension")) -> (w132:dbl[])
      n14 = global write "GVMethodenwechsel.vi" "Methodenwechsel?"(FALSE ("Methodenwechsel?")) -> ()
      n15 = Build Array (concatenate)(w48, w47, w46, w45) -> (w44:dbl[][])
      n16 = Bundle("Modul1/AI sicherer Bereich"=w53, "Modul2/AI sicherer Bereich"=w52, "Modul3/AI sicherer Bereich"=w51, "Traps/Machs sicherer Bereich"=w50, w44, "Metavariablen grüner Bereich"=w43) -> (w49:T18)  [unwired: 1 in]
      n17 = Concatenate Strings("?SE0,SETP,1700" ("string"), "\r\n") -> (w60:string)
      n18 = Concatenate Strings("?SE0,SETP,2200" ("string"), "\r\n") -> (w67:string)
      n19 = String To Byte Array(string=w67) -> (unsigned byte array=w72:u8[])
      n20 = Join Numbers(hi=w72, lo=u8 6) -> ((hi.lo)=w70:u16[])
      n21 = String To Byte Array(string=w60) -> (unsigned byte array=w62:u8[])
      n22 = Join Numbers(hi=w62, lo=u8 5) -> ((hi.lo)=w59:u16[])
      n23 = xnode "Invoke Method"("FPGA VI Reference In"=w57, "Data"=w59) -> ("FPGA VI Reference Out"=w65:refnum<k20>)  [unwired: 2 in, 2 out]
      n24 = xnode "Invoke Method"("FPGA VI Reference In"=w65, "Data"=w70) -> ("FPGA VI Reference Out"=w56:refnum<k20>)  [unwired: 2 in, 2 out]
      n25 = global write "GVProbenvol.vi" "Probenvol.1"(w128) -> ()
      n26 = global write "GVProbenvol.vi" "Probenvol.2"(w128) -> ()
      n27 = global write "GVECDs.vi" "ECD1MW"(w135) -> ()
      n28 = global write "GVECDs.vi" "ECD2MW"(w135) -> ()
      n29 = global write "GVECDs.vi" "ECD1Empfangen?"(w136) -> ()
      n30 = global write "GVECDs.vi" "ECD2Empfangen?"(w136) -> ()
      n31 = property on="dargestellte Größe 2" class="Ring (strict)"("AllowUndefVals"=w232) -> ()  [unwired: 2 in, 2 out]
      n32 = property on="Zeitachse2" class="Ring (strict)"("AllowUndefVals"=w232) -> ()  [unwired: 2 in, 2 out]
      n33 = property on="Zeitachse1" class="Ring (strict)"("AllowUndefVals"=w232) -> ()  [unwired: 2 in, 2 out]
      n34 = property on="dargestellte Größe 1" class="Ring (strict)"("AllowUndefVals"=w232) -> ()  [unwired: 2 in, 2 out]
      n35 = property on="Methode" class="Ring (strict)"("AllowUndefVals"=w232) -> ()  [unwired: 2 in, 2 out]
      n36 = local write "global stop RT"(w233) -> ()
      n37 = global write "gvbooleschRT.vi" "global stop RT"(w233) -> ()
      n38 = global write "GVZeitenZyklen.vi" "ZyklusNummern"(w129) -> ()
      n39 = global write "GVZeitenZyklen.vi" "ZyklusNummernGesamt"(w129) -> ()
      n40 = global write "GVZeitenZyklen.vi" "Big Ben, Methodenzeit, Zykluszeit0, Zykluszeit1, Zykluszeit2A, Zykluszeit2B"(w132) -> ()
      n41 = property on="Methode" class="Ring (strict)"("Value"=w111) -> ()  [unwired: 2 in, 2 out]
      n42 = call "MPVSenden-01-17.vi"("Ventilposition"=0, "FPGA VI Reference In"=w56) -> ("FPGA VI Reference Out"=w54:refnum<k20>)  [unwired: 1 in, 2 out]
      n43 = Initialize Array(-1.0 ("Element"), 6 ("Dimension")) -> (w139:dbl[])
      n44 = Initialize Array(FALSE, 10 ("Dimension")) -> (w147:bool[])
      n45 = Initialize Array(-1.0 ("Element"), 96 ("Dimension")) -> (w140:dbl[])
      n46 = global write "GVZwangs.vi" "ZwangsFPGABoolesch!"(w147) -> ()
      n47 = global write "GVZwangs.vi" "ZwangsFPGABoolesch?"(w147) -> ()
      n48 = global write "GVTrapsMachs.vi" "Traps/Machs"(w139) -> ()
      n49 = global write "GVAIs.vi" "AIs"(w140) -> ()
      n50 = for {
        tunnel: w146 -> [w385] mode=indexing
        tunnel: [w382] -> w145 mode=indexing
        tunnel: [w380] -> w144 mode=indexing
        n51 = Initialize Array(0.0 ("Element"), w385) -> (w383:dbl[])
        n52 = Initialize Array(FALSE, w385) -> (w381:bool[])
        n53 = Bundle(w383) -> (w382:cluster{dbl[]})  [unwired: 1 in]
        n54 = Bundle(w381) -> (w380:cluster{bool[]})  [unwired: 1 in]
      }
      n55 = Bundle("DIOsMod0Name"=w85, "DIOsMod1Name"=w86, "DIOsMod2AName"=w84, "DIOsMod2BName"=w83, "ReglerNameMod0"=w102, "ReglerNameMod1"=w101, "ReglerNameMod2A"=w100, "ReglerNameMod2B"=w99, "LangsameHeizungen"=w173) -> (w235:T19)  [unwired: 1 in]
      n56 = Build Array (concatenate)(w102, w101, w100, w99) -> (w126:string[])
      n57 = Build Array (concatenate)(w195, w194, w193, w192) -> (w246:string[])
      n58 = Build Array (concatenate)(w199, w198, w197, w196) -> (w247:string[])
      n59 = Build Array (concatenate)(w191, w190, w189, w188) -> (w239:dbl[])
      n60 = Build Array (concatenate)(w187, w186, w185, w184) -> (w245:string[])
      n61 = Build Array (concatenate)(w102, w101, w100, w99) -> (→"HorstRegler":string[])
      n62 = Array Size(array=w106) -> (size(s)=w105:i32)
      n63 = Build Array(w156, w155, w154, w153) -> (w152:i32[][])
      n64 = Array Size(array=w173) -> (size(s)=w172:i32)
      n65 = Add Array Elements(numeric array=w146) -> (sum=w231:i32)
      n66 = Array Size(array=w143) -> (size(s)=w142:i32)
      n67 = Index Array(array=w112, index=w111) -> (element=w110:T20)
      n68 = Add Array Elements(numeric array=w146) -> (sum=w158:i32)
      n69 = Build Cluster Array(w156, w155, w154, w153) -> (w238:cluster{"DIOsMod2BNr":i32[]}[])
      n70 = Decrement(x=w168) -> (x-1=w167:i32[])
      n71 = Build Array (concatenate)(w179, w178, w177) -> (w117:string[])
      n72 = Index Array(array=w180, index (col)=0 ("Deaktivierter Index (Spalte)")) -> (element=w225:dbl[])  [unwired: 1 in]
      n73 = Index Array(array=w180, index (col)=1 ("Deaktivierter Index (Spalte)")) -> (element=w226:dbl[])  [unwired: 1 in]
      n74 = Index Array(array=w180, index (col)=2 ("Deaktivierter Index (Spalte)")) -> (element=w227:dbl[])  [unwired: 1 in]
      n75 = for {
        tunnel: w238 -> [w410] mode=indexing
        tunnel: [w411] -> w237 mode=indexing
        n76 = Unbundle(w410) -> ("DIOsMod2BNr"=w409:i32[])
        n77 = Array Size(array=w409) -> (size(s)=w411:i32)
      }
      n78 = property on="Methode" class="Ring (strict)"("Strings []"=w240) -> ()  [unwired: 2 in, 2 out]
      n79 = Build Array (concatenate)(w140, w139) -> (w138:dbl[])
      n80 = Array Size(array=w152) -> (size(s)=w151:i32[])
      n81 = Unbundle(w110) -> ("SPMPV"=w109:i32[])  [unwired: 44 out]
      n82 = Open/Create/Replace File(file path (use dialog)=path "c:/fromcriordy.txt" ("Dateipfad (Dialog verwenden)"), operation (0:open)=T14."replace or create" ("Operation (0:Öffnen)")) -> (refnum out=w204:refnum<file>, error out=w205:errorcluster)  [unwired: 4 in, 1 out]
      n83 = Initialize Array(0.0 ("Element"), w158) -> (w157:dbl[])
      n84 = Initialize Array(0.0 ("element"), w105) -> (w103:dbl[])
      n85 = Get Date/Time In Seconds() -> (seconds since 1Jan1904=w97:timestamp)
      n86 = Initialize Array(FALSE, w142) -> (w137:bool[])
      n87 = Multiply(x=w167, y=32) -> (x*y=w170:i32[])
      n88 = Initialize Array(-1.0, w158) -> (w160:dbl[])
      n89 = Array Subset(array=w117, index=32 ("Index"), length=32 ("Länge")) -> (→"AIs2":string[])
      n90 = Array Subset(array=w117, index=0 ("Index"), length=32 ("Länge")) -> (→"AIs1":string[])
      n91 = Array Subset(array=w117, index=64 ("Index"), length=32 ("Länge")) -> (→"AIs3":string[])
      n92 = global write "GVZwangs.vi" "ZwangsLangsameHeizungenAn!"(w137) -> ()
      n93 = global write "GVZwangs.vi" "ZwangsLangsameHeizungenAn?"(w137) -> ()
      n94 = global write "GVHK1Hz.vi" "Mod1Mod2Mod3/AITrapsMachs1Hz"(w138) -> ()
      n95 = global write "GVHorstSP.vi" "HorstSP"(w157) -> ()
      n96 = for {
        tunnel: w151 -> [w390] mode=indexing
        tunnel: [w387] -> w150 mode=indexing
        n97 = Initialize Array(FALSE, w390) -> (w388:bool[])
        n98 = Bundle(w388) -> (w387:cluster{bool[]})  [unwired: 1 in]
      }
      n99 = global write "GVMetavariablen.vi" "Metavariablen"(w103) -> ()
      n100 = global write "GVHeizenLH.vi" "Heizen?LH"(w137) -> ()
      n101 = Add(x=w170, y=w143) -> (x+y=w169:i32[])
      n102 = Close File(refnum=w204, error in=w205) -> (path=w236:path)  [unwired: 1 out]
      n103 = Format Date/Time String(time format string (%c)="%Y-%m-%d--%H-%M" ("Zeitformatierungs-String (%c)"), seconds (now)=w97) -> (date/time string=w75:string)  [unwired: 1 in]
      n104 = Index Array(array=w109, index=0) -> (element=w107:i32)
      n105 = global write "GVMWHorst.vi" "MWHorst"(w160) -> ()
      n106 = global write "GVVentilposition.vi" "Ventilposition"(w107) -> ()
      n107 = Build Array (concatenate)(string[] ["Jahr", "Monat", "Tag", "Stunde", "Minute", "Sekunde"] ("Array"), string[] ["Datei Nr.", "Methode Nr.", "Zyklusnr. Mod0", "Zyklusnr. Mod1", "Zyklusnr. Mod2A", "Zyklusnr. Mod2B"], w242, w117, w127, w126, "Probenvolumen1", "Probenvolumen2", "Ventilposition" ("element"), string[] ["CPU Total", "CPU Time critical", "CPU Timed Structures", "CPU High", "CPU Above normal", "CPU Normal", "CPU Background", "CPU Idle", "CPU ISR", "Memory", "SekundenTotalBrutal"]) -> (w244:string[])
      n108 = Build Array (concatenate)(w127, w126) -> (w125:string[])
      n109 = Build Array (concatenate)(w117, w127, w126) -> (w124:string[])
      n110 = Split 1D Array(array=w242, index=2 ("Index")) -> (second subarray=w234:string[])  [unwired: 1 out]
      n111 = Concatenate Strings("HK " ("String"), w75) -> (w79:string)
      n112 = Concatenate Strings("ECD1 " ("String"), w75) -> (w77:string)
      n113 = Concatenate Strings("ECD2 " ("String"), w75) -> (w74:string)
      n114 = property on="dargestellte Größe 1" class="Ring (strict)"("Strings []"=w124) -> ()  [unwired: 2 in, 2 out]
      n115 = property on="Zeitachse2" class="Ring (strict)"("Strings []"=w234) -> ()  [unwired: 2 in, 2 out]
      n116 = property on="Zeitachse1" class="Ring (strict)"("Strings []"=w234) -> ()  [unwired: 2 in, 2 out]
      n117 = property on="dargestellte Größe 3" class="Ring (strict)"("Strings []"=w125) -> ()  [unwired: 2 in, 2 out]
      n118 = global write "GVZwangs.vi" "ZwangsHorst!"(w145) -> ()
      n119 = property on="dargestellte Größe 2" class="Ring (strict)"("Strings []"=w124) -> ()  [unwired: 2 in, 2 out]
      n120 = global write "GVZwangs.vi" "ZwangsHorst?"(w144) -> ()
      n121 = Build Path(base path=w82, name or relative path=w79) -> (appended path=w90:path)
      n122 = Build Path(base path=w96, name or relative path=w77) -> (appended path=w92:path)
      n123 = Build Path(base path=w95, name or relative path=w74) -> (appended path=w94:path)
      n124 = Create Folder(path (use dialog)=w90) -> (created path=w89:path)  [unwired: 2 in, 2 out]
      n125 = Create Folder(path (use dialog)=w92) -> (created path=w91:path)  [unwired: 2 in, 2 out]
      n126 = Create Folder(path (use dialog)=w94) -> (created path=w93:path)  [unwired: 2 in, 2 out]
      n127 = global write "GVZwangs.vi" "ZwangsDIO!"(w150) -> ()
      n128 = global write "GVZwangs.vi" "ZwangsDIO?"(w150) -> ()
      n129 = case shown="True" w113 {
        tunnel: [w401 w406] -> w218
        tunnel: [w401 w405] -> w217
        tunnel: w89 -> [_ w404]
        tunnel: w176 -> [_ w403]
        tunnel: w111 -> [_ w402]
        frame False {
          w401 = refnum<k34> refnum ("tdms1")
        }
        frame True {
          n130 = call "TDMS0.vi"("Startmethode"=w402, "Dateiname"=w403, "Dateiordner"=w404) -> ("tdms1"=w405:refnum<k34>, "tdms0"=w406:refnum<k34>)
          n131 = global write "GVaktuelleTDMS.vi" "aktuelleTDMS-DateiHK"(w406) -> ()
        }
      }
      n132 = case shown="True" w113 {
        tunnel: [w391 w400] -> w216
        tunnel: [w391 w399] -> w215
        tunnel: [w391 w398] -> w214
        tunnel: [w391 w397] -> w213
        tunnel: w91 -> [_ w396]
        tunnel: w175 -> [_ w395]
        tunnel: w93 -> [_ w394]
        tunnel: w174 -> [_ w393]
        tunnel: w111 -> [_ w392]
        frame False {
          w391 = refnum<k34> refnum ("tdms0")
        }
        frame True {
          n133 = call "TDMS0.vi"("Startmethode"=w392, "Dateiname"=w395, "Dateiordner"=w396) -> ("tdms1"=w399:refnum<k34>, "tdms0"=w400:refnum<k34>)
          n134 = call "TDMS0.vi"("Startmethode"=w392, "Dateiname"=w393, "Dateiordner"=w394) -> ("tdms1"=w397:refnum<k34>, "tdms0"=w398:refnum<k34>)
          n135 = global write "GVaktuelleTDMS.vi" "aktuelleTDMS-DateiECD1"(w400) -> ()
          n136 = global write "GVaktuelleTDMS.vi" "aktuelleTDMS-DateiECD2"(w398) -> ()
        }
      }
      n137 = Open/Create/Replace File(file path (use dialog)=path "c:/fromcriocmd.txt" ("Pfad MS-Datei CRIO"), operation (0:open)=T14."replace or create" ("Operation (0:Öffnen)")) -> (refnum out=w210:refnum<file>, error out=w209:errorcluster)  [unwired: 4 in, 1 out]
      n138 = call "AIKoeffSortieren.vi"("Modul3/AI koeff"=w181, "Modul2/AI koeff"=w182, "Modul1/AI koeff"=w183) -> ("P0"=w222:dbl[], "P1"=w223:dbl[], "P2"=w224:dbl[])
      n139 = Write to Text File(file (use dialog)=w210, text="time=yyyymmddhhmmss\ncycle=005\ninfo=1234567890123456789012345678901234567890123456789012345678901234567890123456789012345678901234567890\nlength=100\ncmd=cycle" ("Text0 MS-Datei"), error in=w209) -> (refnum out=w207:refnum<file>, error out=w206:errorcluster)  [unwired: 1 in, 1 out]
      n140 = Bundle("created path"=w89, "created path"=w91, "created path"=w93, "Dateiname Housekeeping"=w176, "DateinameECD1"=w175, "DateinameECD2"=w174, "tdms0"=w218, "tdms1"=w217, "tdms0"=w216, "tdms1"=w215, "tdms0"=w214, "tdms1"=w213) -> (w219:T21)  [unwired: 1 in]
      n141 = Close File(refnum=w207, error in=w206) -> (path=w201:path)  [unwired: 1 out]
      "schnelle Heizungen" <- string[] ["Trap1 [°C]", "Trap2 [°C]", "PreCol1 [°C]", "PreCol2 [°C]", "MainCol1 [°C]", "MainCol2 [°C]"]
    }
    frame #1 {
      w420 = dbl[] [-1.0]
      w491 = 0
      w466 = 0 ("Zyklusnummer1")
      n142 = while {
        tunnel: w444 -> [w873]
        tunnel: w513 -> [w872]
        tunnel: w512 -> [w871]
        tunnel: w511 -> [w870]
        shift-right: [w869] -> _
        shift-left: errorcluster {"status"=FALSE, "code"=0, "source"=""} ("error out") -> [w868]
        stop <- w874 stop-if-true
        n143 = call "AIsFIFORT-01-17.vi"("FPGA VI Reference In"=w873, "P2"=w872, "P1"=w871, "P0"=w870, "error in"=w868) -> ("error out"=w869:errorcluster)
        "AIsFIFOread" <- w869
        n144 = global read "gvbooleschRT.vi" "global stop RT"() -> (w874:bool)
      }
      n145 = Add Array Elements(numeric array=w440) -> (sum=w439:i32)
      n146 = Array Size(array=w448) -> (size(s)=w469:i32)
      n147 = Unbundle(w465) -> ("created path"=w464:path, "created path"=w462:path, "created path"=w461:path, "Dateiname Housekeeping"=w463:string, "DateinameECD1"=w460:string, "DateinameECD2"=w459:string, "tdms0"=w458:refnum<k34>, "tdms1"=w457:refnum<k34>, "tdms0"=w456:refnum<k34>, "tdms1"=w455:refnum<k34>, "tdms0"=w454:refnum<k34>, "tdms1"=w453:refnum<k34>)
      n148 = while {
        stop <- w1316 stop-if-true
        w1310 = 10.0
        n149 = call "Warten2"("Count(mSec)"=u32 1000) -> ()  [unwired: 1 out]
        n150 = global read "gvbooleschRT.vi" "global stop RT"() -> (w1316:bool)
        n151 = global read "GVTrapsMachs.vi" "Traps/Machs"() -> (w1306:dbl[])
        n152 = global read "GVAIs.vi" "AIs"() -> (w1307:dbl[])
        n153 = for {
          N: 9 -> [_]
          shift-right: [w1319] -> w1313
          shift-left: w1307 -> [w1320]
          shift-right: [w1317] -> w1311
          shift-left: w1306 -> [w1318]
          n154 = flat-sequence {
            tunnel: w1320 -> [w1327]
            tunnel: [w1326] -> w1319
            tunnel: w1318 -> [w1325]
            tunnel: [w1324] -> w1317
            frame #0 {
              n155 = call "Warten28"("Count(mSec)"=u32 100) -> ()  [unwired: 1 out]
            }
            frame #1 {
              n156 = global read "GVAIs.vi" "AIs"() -> (w1323:dbl[])
              n157 = Add(x=w1327, y=w1323) -> (x+y=w1326:dbl[])
              n158 = global read "GVTrapsMachs.vi" "Traps/Machs"() -> (w1322:dbl[])
              n159 = Add(x=w1322, y=w1325) -> (x+y=w1324:dbl[])
            }
          }
        }
        n160 = Divide(x=w1313, y=w1310) -> (x/y=w1312:dbl[])
        n161 = Divide(x=w1311, y=w1310) -> (x/y=w1309:dbl[])
        n162 = Build Array (concatenate)(w1312, w1309) -> (w1308:dbl[])
        n163 = global write "GVHK1Hz.vi" "Mod1Mod2Mod3/AITrapsMachs1Hz"(w1308) -> ()
      }
      n164 = while {
        shift-right: ["Methode"] -> _
        shift-left: w517 -> [w1330]
        stop <- w1332 stop-if-true
        n165 = call "Bis zum nächsten Vielfachen warten7"("Count(mSec)"=u32 1000) -> ()  [unwired: 1 out]
        n166 = Not Equal?(x=w1330, y="Methode") -> (x != y?=w1328:bool)
        n167 = global write "GVMethodenwechsel.vi" "Methodenwechsel?"(w1328) -> ()
        n168 = global read "gvbooleschRT.vi" "global stop RT"() -> (w1332:bool)
      }
      n169 = Index Array(array=w441, index #1=0 ("Index"), index #2=1 ("Index"), index #3=2 ("Index"), index #4=3 ("Index")) -> (element #1=w480:i32, element #2=w479:i32, element #3=w482:i32, element #4=w481:i32)
      n170 = while {
        tunnel: w444 -> [w875]
        tunnel: w419 -> [w880]
        tunnel: w418 -> [w879]
        tunnel: w417 -> [w878]
        shift-right: [w877] -> _
        shift-left: errorcluster {"status"=FALSE, "code"=0, "source"=""} ("error out") -> [w876]
        stop <- w882 stop-if-true
        n171 = call "TrapsMachMitteln-01-17.vi"("FPGA VI Reference In"=w875, "Traps/MachKoeff2"=w880, "Traps/MachKoeff1"=w879, "Traps/MachKoeff0"=w878, "error in"=w876) -> ("error out"=w877:errorcluster)
        "MWTrapsMachs" <- w877
        n172 = global read "gvbooleschRT.vi" "global stop RT"() -> (w882:bool)
        n173 = call "Bis zum nächsten Vielfachen warten16"("Count(mSec)"=u32 100) -> ()  [unwired: 1 out]
      }
      n174 = call <vilib>:"Space Constant.vi"() -> ("String"=w426:string)
      n175 = case shown="True" TRUE ("ECDSpeichern") {
        frame False {
        }
        frame True {
          w808 = dbl[] []
          n176 = global read "GVaktuelleTDMS.vi" "aktuelleTDMS-DateiECD1"() -> (w809:refnum<k34>)
          n177 = while {
            shift-right: [w821] -> _
            shift-left: w808 -> [w825]
            shift-right: [w814] -> _
            shift-left: w808 -> [w818]
            shift-right: [w820] -> _
            shift-left: w809 -> [w823]
            tunnel: w808 -> [w817]
            shift-right: [w811] -> _
            shift-left: errorcluster {"status"=FALSE, "code"=0, "source"=""} ("error IO") -> [w810]
            stop <- w830 stop-if-true
            n178 = global read "GVaktuelleTDMS.vi" "aktuelleTDMS-DateiECD1"() -> (w820:refnum<k34>)
            n179 = global read "GVaktuelleTDMS.vi" "aktuelleTDMS-DateiECD2"() -> (w828:refnum<k34>)
            n180 = call "Bis zum nächsten Vielfachen warten3"("Count(mSec)"=u32 500) -> ()  [unwired: 1 out]
            n181 = global read "GVECDs.vi" "ECD1MW"() -> (w824:dbl[])
            n182 = global read "GVECDs.vi" "ECD2MW"() -> (w815:dbl[])
            n183 = Equal?(x=w823, y=w820) -> (x = y?=w816:bool)
            n184 = Build Array (concatenate)(w825, w824) -> (w822:dbl[])
            n185 = Build Array (concatenate)(w818, w815) -> (w819:dbl[])
            n186 = TDMS Write(0:w820, 7:"ECD1", 9:w824, 11:w810) -> (15:w813:errorcluster)  [unwired: 2 in, 3 out]
            n187 = TDMS Write(0:w828, 7:"ECD2", 9:w815, 11:w810) -> (15:w812:errorcluster)  [unwired: 2 in, 3 out]
            n188 = Select(t=w819, s=w816, f=w817) -> (s? t:f=w814:dbl[])
            n189 = Select(t=w822, s=w816, f=w817) -> (s? t:f=w821:dbl[])
            n190 = Merge Errors(w813, w812) -> (w811:errorcluster)
            "TDMSwriteECD" <- w811
            n191 = global write "GVChroms.vi" "ECD2Chrom"(w814) -> ()
            n192 = global write "GVChroms.vi" "ECD1Chrom"(w821) -> ()
            n193 = global read "gvbooleschRT.vi" "global stop RT"() -> (w830:bool)
          }
        }
      }
      n194 = while {
        shift-right: [w524] -> _
        shift-left: w420 -> [w526]
        shift-right: [w523] -> _
        shift-left: w420 -> [w525]
        stop <- w528 stop-if-true
        n195 = call "Bis zum nächsten Vielfachen warten"("Count(mSec)"=u32 100) -> ()  [unwired: 1 out]
        n196 = case shown="True" "An/Aus" {
          tunnel: w526 -> [w530 w546]
          tunnel: w525 -> [w529 w545]
          tunnel: [w530 w539] -> w524
          tunnel: [w529 w538] -> w523
          frame False {
          }
          frame True {
            w542 = dbl[] [] ("t")
            n197 = global read "GVMWHorst.vi" "MWHorst"() -> (w535:dbl[])
            n198 = global read "GVTrapsMachs.vi" "Traps/Machs"() -> (w536:dbl[])
            n199 = Build Array (concatenate)(w536, w535) -> (w534:dbl[])
            n200 = Index Array(array=w534, index="dargestellte Größe 3") -> (element=w547:dbl)
            n201 = Build Array (concatenate)(w546, w547) -> (w540:dbl[])
            n202 = Select(t=w542, s="TafelWischen!", f=w540) -> (s? t:f=w539:dbl[])
            n203 = global read "GVZeitenZyklen.vi" "Big Ben, Methodenzeit, Zykluszeit0, Zykluszeit1, Zykluszeit2A, Zykluszeit2B"() -> (w533:dbl[])
            n204 = Index Array(array=w533, index=1 ("Index")) -> (element=w531:dbl)
            n205 = Build Array (concatenate)(w545, w531) -> (w541:dbl[])
            n206 = Select(t=w542, s="TafelWischen!", f=w541) -> (s? t:f=w538:dbl[])
            n207 = Bundle(w541, w540) -> (→"schnelleAnzeige":cluster{dbl[], dbl[]})  [unwired: 1 in]
          }
        }
        n208 = global read "gvbooleschRT.vi" "global stop RT"() -> (w528:bool)
      }
      n209 = case shown="True" TRUE ("HKSpeichern") {
        tunnel: w515 -> [_ w861]
        frame False {
        }
        frame True {
          n210 = while {
            tunnel: w861 -> [w865]
            shift-right: [w863] -> _
            shift-left: errorcluster {"status"=FALSE, "code"=0, "source"=""} ("error out") -> [w862]
            stop <- w867 stop-if-true
            n211 = local read "Methode"() -> (w864:i32)
            n212 = call "Bis zum nächsten Vielfachen warten2"("Count(mSec)"=u32 1000) -> ()  [unwired: 1 out]
            n213 = call "HKinTDMS-01-16.vi"("Methode"=w864, "error in (no error)"=w862, "Kanäle"=w865) -> ("error out"=w863:errorcluster)
            "TDMSwriteHK" <- w863
            n214 = global read "gvbooleschRT.vi" "global stop RT"() -> (w867:bool)
          }
        }
      }
      n215 = for {
        N: 1 -> [_]
        tunnel: w444 -> [w883]
        tunnel: [w883] -> w471
        n216 = call "Warten8"("Count(mSec)"=u32 100) -> ()  [unwired: 1 out]
      }
      n217 = global read "GVVentilposition.vi" "Ventilposition"() -> (w450:i32)
      n218 = Build Array(w426) -> (w425:string[])
      n219 = Initialize Array(-1 ("Element"), 4 ("Dimension")) -> (w442:i32[])
      n220 = case shown="True" TRUE {
        tunnel: w466 -> [_ w840]
        tunnel: w464 -> [_ w839]
        tunnel: w463 -> [_ w838]
        tunnel: w458 -> [_ w837]
        tunnel: w457 -> [_ w836]
        frame False {
        }
        frame True {
          w831 = errorcluster {"status"=FALSE, "code"=0, "source"=""} ("error out TDMSopen")
          n221 = while {
            shift-right: [w845] -> w835
            shift-left: w837 -> [w847]
            shift-right: [w856] -> w834
            shift-left: w836 -> [w849]
            shift-right: [w851] -> _
            shift-left: w840 -> [w857]
            tunnel: w838 -> [w853]
            tunnel: w839 -> [w854]
            shift-right: [w844] -> w833
            shift-left: w831 -> [w842]
            shift-right: [w843] -> w832
            shift-left: w831 -> [w841]
            stop <- w859 stop-if-true
            n222 = global read "GVZeitenZyklen.vi" "ZyklusNummernGesamt"() -> (w846:i32[])
            n223 = call "Bis zum nächsten Vielfachen warten5"("Count(mSec)"=u32 500) -> ()  [unwired: 1 out]
            n224 = Index Array(array=w846, index=1 ("Index")) -> (element=w851:i32)
            n225 = Greater?(x=w851, y=w857) -> (0:w850:bool)
            n226 = Select(t=w849, s=w850, f=w847) -> (s? t:f=w848:refnum<k34>)
            n227 = local read "Methode"() -> (w855:i32)
            n228 = global write "GVaktuelleTDMS.vi" "aktuelleTDMS-DateiHK"(w848) -> ()
            n229 = call "AktuelleTDMS.vi"("AktuelleTDMS"=w847, "error in TDMSopen"=w842, "Dateiordner"=w854, "NächsteTDMS"=w849, "NeuerZyklus?"=w850, "Methodennummer"=w855, "Zyklnumges"=w851, "error in TDMSclose"=w841, "Dateiname"=w853) -> ("AktuelleTDMS"=w845:refnum<k34>, "error out TDMSopen"=w844:errorcluster, "error out TDMSclose"=w843:errorcluster, "NächsteTDMS"=w856:refnum<k34>)  [unwired: 3 in]
            "TDMSopenHK" <- w844
            "TDMScloseHK" <- w843
            n230 = global read "gvbooleschRT.vi" "global stop RT"() -> (w859:bool)
          }
          n231 = TDMS Close(8:w833, 11:w835) -> ()  [unwired: 2 out]
          n232 = TDMS Close(8:w832, 11:w834) -> ()  [unwired: 2 out]
        }
      }
      n233 = case shown="True" TRUE {
        tunnel: w466 -> [_ w768]
        tunnel: w462 -> [_ w767]
        tunnel: w461 -> [_ w766]
        tunnel: w460 -> [_ w765]
        tunnel: w459 -> [_ w764]
        tunnel: w456 -> [_ w763]
        tunnel: w455 -> [_ w762]
        tunnel: w454 -> [_ w761]
        tunnel: w453 -> [_ w760]
        frame False {
        }
        frame True {
          w753 = errorcluster {"status"=FALSE, "code"=0, "source"=""} ("error out TDMSopen")
          n234 = while {
            shift-right: [w792] -> w759
            shift-left: w763 -> [w794]
            shift-right: [w802] -> w758
            shift-left: w762 -> [w796]
            shift-right: [w800] -> _
            shift-left: w768 -> [w803]
            tunnel: w767 -> [w799]
            tunnel: w765 -> [w798]
            shift-right: [w791] -> w754
            shift-left: w753 -> [w789]
            shift-right: [w790] -> w755
            shift-left: w753 -> [w788]
            stop <- w805 stop-if-true
            n235 = global read "GVZeitenZyklen.vi" "ZyklusNummernGesamt"() -> (w793:i32[])
            n236 = call "Bis zum nächsten Vielfachen warten4"("Count(mSec)"=u32 500) -> ()  [unwired: 1 out]
            n237 = Index Array(array=w793, index=2 ("Index")) -> (element=w800:i32)
            n238 = Greater?(x=w800, y=w803) -> (0:w797:bool)
            n239 = Select(t=w796, s=w797, f=w794) -> (s? t:f=w795:refnum<k34>)
            n240 = local read "Methode"() -> (w801:i32)
            n241 = global write "GVaktuelleTDMS.vi" "aktuelleTDMS-DateiECD1"(w795) -> ()
            n242 = call "AktuelleTDMS.vi"("AktuelleTDMS"=w794, "error in TDMSopen"=w789, "Dateiordner"=w799, "NächsteTDMS"=w796, "NeuerZyklus?"=w797, "Methodennummer"=w801, "Zyklnumges"=w800, "error in TDMSclose"=w788, "Dateiname"=w798) -> ("AktuelleTDMS"=w792:refnum<k34>, "error out TDMSopen"=w791:errorcluster, "error out TDMSclose"=w790:errorcluster, "NächsteTDMS"=w802:refnum<k34>)  [unwired: 3 in]
            "TDMSopenECD1" <- w791
            "TDMScloseECD1" <- w790
            n243 = global read "gvbooleschRT.vi" "global stop RT"() -> (w805:bool)
          }
          n244 = while {
            shift-right: [w782] -> w757
            shift-left: w761 -> [w774]
            shift-right: [w783] -> w756
            shift-left: w760 -> [w776]
            shift-right: [w780] -> _
            shift-left: w768 -> [w784]
            tunnel: w766 -> [w779]
            tunnel: w764 -> [w778]
            shift-right: [w772] -> _
            shift-left: w753 -> [w770]
            shift-right: [w771] -> _
            shift-left: w753 -> [w769]
            stop <- w786 stop-if-true
            n245 = global read "GVZeitenZyklen.vi" "ZyklusNummernGesamt"() -> (w773:i32[])
            n246 = call "Bis zum nächsten Vielfachen warten6"("Count(mSec)"=u32 500) -> ()  [unwired: 1 out]
            n247 = Index Array(array=w773, index=3 ("Index")) -> (element=w780:i32)
            n248 = Greater?(x=w780, y=w784) -> (0:w777:bool)
            n249 = Select(t=w776, s=w777, f=w774) -> (s? t:f=w775:refnum<k34>)
            n250 = local read "Methode"() -> (w781:i32)
            n251 = global write "GVaktuelleTDMS.vi" "aktuelleTDMS-DateiECD2"(w775) -> ()
            n252 = call "AktuelleTDMS.vi"("AktuelleTDMS"=w774, "error in TDMSopen"=w770, "Dateiordner"=w779, "NächsteTDMS"=w776, "NeuerZyklus?"=w777, "Methodennummer"=w781, "Zyklnumges"=w780, "error in TDMSclose"=w769, "Dateiname"=w778) -> ("AktuelleTDMS"=w782:refnum<k34>, "error out TDMSopen"=w772:errorcluster, "error out TDMSclose"=w771:errorcluster, "NächsteTDMS"=w783:refnum<k34>)  [unwired: 3 in]
            "TDMSopenECD2" <- w772
            "TDMScloseECD2" <- w771
            n253 = global read "gvbooleschRT.vi" "global stop RT"() -> (w786:bool)
          }
          n254 = TDMS Close(8:w754, 11:w759) -> ()  [unwired: 2 out]
          n255 = TDMS Close(8:w755, 11:w758) -> ()  [unwired: 2 out]
          n256 = TDMS Close(11:w757) -> ()  [unwired: 1 in, 2 out]
          n257 = TDMS Close(11:w756) -> ()  [unwired: 1 in, 2 out]
        }
      }
      n258 = Add(x=w482, y=w481) -> (x+y=w478:i32)
      n259 = Bundle(w425, w425, w425) -> (w489:cluster{string[], string[], string[]})  [unwired: 1 in]
      n260 = Index Array(array=w435, index=w433) -> (element=w434:T20)
      n261 = Initialize Array(cluster{"output high":dbl, "output low":dbl} {"output high"=99999.0, "output low"=0.0} ("output range"), w469) -> (w449:cluster{"output high":dbl, "output low":dbl}[])
      n262 = Concatenate Strings("?SE0,GDATA" ("Schreibpuffer"), "\r") -> (w421:string)
      n263 = Build Array(w480, w479, w478) -> (w477:i32[])
      n264 = while {
        tunnel: w516 -> [w1010]
        shift-right: [w1009] -> _
        shift-left: w435 -> [w991]
        tunnel: w449 -> [w1008]
        tunnel: w448 -> [w1007]
        tunnel: w444 -> [w1006]
        tunnel: w447 -> [w1005]
        tunnel: w446 -> [w1004]
        shift-right: [w998] -> _
        shift-left: 0 -> [w1003]
        tunnel: w444 -> [w1002]
        tunnel: w443 -> [w1001]
        shift-right: [w997] -> _
        shift-left: w442 -> [w1000]
        tunnel: w441 -> [w992]
        tunnel: w440 -> [w993]
        tunnel: w439 -> [w994]
        tunnel: w438 -> [w995]
        tunnel: w437 -> [w996]
        tunnel: w436 -> [w999]
        shift-right: [w914] -> _
        shift-left: w434 -> [w913]
        tunnel: w419 -> [w892]
        tunnel: w418 -> [w896]
        tunnel: w417 -> [w902]
        tunnel: w412 -> [w885]
        i -> [w917]
        stop <- w1011 stop-if-true
        w903 = 0  # ZeileMainMach2
        w904 = 0  # ZeileMainMach1
        w959 = FALSE
        w958 = 0.0
        w960 = 0  # ZeilennummerMPV
        w964 = cluster{dbl[], dbl[]} {[], []}
        w973 = dbl[] []
        w977 = 0  # ZeilePreMach2
        w978 = 0  # ZeilePreMach1
        w979 = 0  # ZeileFPGAFixp
        w980 = 0  # ZeileFPGAPID
        w981 = 0  # ZeileFPGABoolesch
        w982 = i32[] [0, 0, 0, 0]  # ZeilennummernHorst
        w983 = i32[] [0, 0, 0, 0]  # ZeilennummernDIOs
        n265 = Unbundle(w913) -> ("Zykluslängen [s]"=w957:dbl[], "ZeitpktDIOsMod0"=w956:dbl[], "ZeitpktDIOsMod1"=w955:dbl[], "ZeitpktDIOsMod2A"=w954:dbl[], "ZeitpktDIOsMod2B"=w953:dbl[], "DIOsSPMod0"=w952:bool[][], "DIOsSPMod1"=w951:bool[][], "DIOsSPMod2A"=w950:bool[][], "DIOsSPMod2B"=w949:bool[][], "Mod0HorstZeitpkt"=w948:dbl[], "Mod1HorstZeitpkt"=w947:dbl[], "Mod2AHorstZeitpkt"=w946:dbl[], "Mod2BHorstZeitpkt"=w945:dbl[], "HorstSPMod0"=w944:dbl[][], "HorstSPMod1"=w943:dbl[][], "HorstSPMod2A"=w942:dbl[][], "HorstSPMod2B"=w941:dbl[][], "LHSetpoints"=w940:dbl[], "LHHeizen?"=w939:bool[], "ZPktFPGABoolesch"=w938:dbl[], "FPGABoolesch"=w937:bool[][], "ZeitpktFPGAPID"=w936:dbl[], "FPGAPID"=w935:T22, "ZeitpktFPGAFixp"=w934:dbl[], "SHSetpoints"=w933:dbl[][], "t_PreMach1"=w932:dbl[], "T_PreMach1"=w931:dbl[], "t_PreMach2"=w930:dbl[], "T_PreMach2"=w929:dbl[], "PIDs für \"träge\" Heizungen"=w928:T23, "Zwangsbedingungen"=w927:dbl[][], "Dateien fürs MS schicken?"=w926:bool, "ZeitpunkteMPV"=w925:dbl[], "SPMPV"=w924:i32[], "ZeitpktMS-1"=w923:dbl, "ZeitpktMS-2"=w922:dbl, "Int.Start1"=w921:dbl, "Int.Stop1"=w920:dbl, "Int.Start2"=w919:dbl, "Int.Stop2"=w918:dbl, "t_MainMach1"=w912:dbl[], "T_MainMach1"=w911:dbl[], "t_MainMach2"=w910:dbl[], "T_MainMach2"=w909:dbl[])  [unwired: 1 out]
        n266 = Add(x=w1000, y=1) -> (x+y=w968:i32[])
        n267 = Array Subset(array=w902, index=2 ("Index"), length=4 ("Länge")) -> (w899:dbl[])
        n268 = Array Subset(array=w896, index=2 ("Index"), length=4 ("Länge")) -> (w895:dbl[])
        n269 = Array Subset(array=w892, index=2 ("Index"), length=4 ("Länge")) -> (w891:dbl[])
        n270 = local read "Methode"() -> (w916:i32)
        n271 = while {
          tunnel: w993 -> [w1084]
          tunnel: w996 -> [w1082]
          tunnel: w995 -> [w1081]
          tunnel: w992 -> [w1083]
          tunnel: w994 -> [w1080]
          tunnel: w927 -> [w1072]
          stop <- w1074 stop-if-true
          n272 = call "Bis zum nächsten Vielfachen warten10"("Count(mSec)"=u32 1000) -> ()  [unwired: 1 out]
          n273 = local read "Methode"() -> (w1079:i32)
          n274 = global read "GVMethodenwechsel.vi" "Methodenwechsel?"() -> (w1076:bool)
          n275 = global read "gvbooleschRT.vi" "global stop RT"() -> (w1077:bool)
          n276 = case shown="True" "global stop RT" {
            frame False {
            }
            frame True {
              n277 = global write "gvbooleschRT.vi" "global stop RT"(TRUE ("global stop RT")) -> ()
            }
          }
          n278 = call "ZwangsbedingungenGV.vi"("AnzahlHorst"=w1082, "AnzahlHorst/Modul"=w1083, "AnzahlLH"=w1081, "AnzahlDIOs/Modul"=w1084, "AnzahlDIOs"=w1080, "Zwangsbedingungen"=w1072, "Methodennummer"=w1079) -> ("Methodennummer"=w1078:i32)  [unwired: 4 in]
          n279 = local write "Methode"(w1078) -> ()
          n280 = local read "veränderte Methode benutzen"() -> (w1075:bool)
          n281 = Compound Arithmetic op=OR(w1077, w1076, w1075) -> (w1074:bool)
        }
        n282 = while {
          tunnel: w1007 -> [w1063]
          tunnel: w1008 -> [w1065]
          tunnel: w1006 -> [w1060]
          tunnel: w940 -> [w1064]
          tunnel: w928 -> [w1066]
          shift-right: [w1062] -> _
          shift-left: errorcluster {"status"=FALSE, "code"=0, "source"=""} ("error out") -> [w1061]
          stop <- w1067 stop-if-true
          n283 = call "LH-01-17.vi"("FPGA VI Reference In"=w1060, "OutputRange"=w1065, "LHSetpoints"=w1064, "AIsLH"=w1063, "error in"=w1061, "PIDs für \"träge\" Heizungen"=w1066) -> ("error out"=w1062:errorcluster)  [unwired: 1 in]
          "LH" <- w1062
          n284 = call "Bis zum nächsten Vielfachen warten12"("Count(mSec)"=u32 100) -> ()  [unwired: 1 out]
          n285 = local read "veränderte Methode benutzen"() -> (w1068:bool)
          n286 = global read "GVMethodenwechsel.vi" "Methodenwechsel?"() -> (w1069:bool)
          n287 = global read "gvbooleschRT.vi" "global stop RT"() -> (w1070:bool)
          n288 = Compound Arithmetic op=OR(w1070, w1069, w1068) -> (w1067:bool)
        }
        n289 = Build Cluster Array(w952, w951, w950, w949) -> (w987:cluster{"DIOsSPMod2B":bool[][]}[])
        n290 = Build Cluster Array(w944, w943, w942, w941) -> (w985:cluster{"HorstSPMod2B":dbl[][]}[])
        n291 = Build Cluster Array(w956, w955, w954, w953) -> (w988:cluster{"ZeitpktDIOsMod2B":dbl[]}[])
        n292 = Build Cluster Array(w948, w947, w946, w945) -> (w986:cluster{"Mod2BHorstZeitpkt":dbl[]}[])
        n293 = Bundle(w899, w895, w891) -> (w890:cluster{dbl[], dbl[], dbl[]})  [unwired: 1 in]
        n294 = Equal?(x=w917, y=0) -> (x = y?=w989:bool)
        n295 = global read "GVZeitenZyklen.vi" "ZyklusNummern"() -> (w967:i32[])
        n296 = global read "GVZwangs.vi" "ZwangsHorst?"() -> (w972:cluster{bool[]}[])
        n297 = global read "gvbooleschRT.vi" "global stop RT"() -> (w1011:bool)
        n298 = global read "GVZwangsMPV.vi" "ZwangsMPV?"() -> (w888:bool)
        n299 = global read "GVZwangs.vi" "ZwangsDIO?"() -> (w971:cluster{bool[]}[])
        n300 = global read "GVaktuelleTDMS.vi" "aktuelleTDMS-DateiECD1"() -> (w966:refnum<k34>)
        n301 = global read "GVZwangs.vi" "ZwangsFPGABoolesch?"() -> (w970:bool[])
        n302 = while {
          shift-right: [w1024] -> _
          shift-left: w959 -> [w1028]
          shift-right: [w1023] -> _
          shift-left: w958 -> [w1027]
          shift-right: [w1022] -> _
          shift-left: w959 -> [w1026]
          shift-right: [w1021] -> _
          shift-left: w958 -> [w1025]
          tunnel: w999 -> [w1020]
          tunnel: w921 -> [w1015]
          tunnel: w920 -> [w1014]
          tunnel: w919 -> [w1013]
          tunnel: w918 -> [w1012]
          stop <- w1017 stop-if-true
          n303 = call "Integrieren.vi"("Integrieren1"=w1028, "Integral1"=w1027, "Integrieren2"=w1026, "Integral2"=w1025, "Int.Start1"=w1015, "Int.Stop1"=w1014, "Int.Start2"=w1013, "HorstProbenflußNr."=w1020, "Int.Stop2"=w1012) -> ("Integrieren1"=w1024:bool, "Integral1"=w1023:dbl, "Integrieren2"=w1022:bool, "Integral2"=w1021:dbl)  [unwired: 7 in]
          n304 = call "Bis zum nächsten Vielfachen warten9"("Count(mSec)"=u32 100) -> ()  [unwired: 1 out]
          n305 = global read "GVMethodenwechsel.vi" "Methodenwechsel?"() -> (w1018:bool)
          n306 = global read "gvbooleschRT.vi" "global stop RT"() -> (w1019:bool)
          n307 = local read "veränderte Methode benutzen"() -> (w1016:bool)
          n308 = Compound Arithmetic op=OR(w1019, w1018, w1016) -> (w1017:bool)
        }
        n309 = while "Zeit" {
          tunnel: w989 -> [w1267]
          tunnel: w957 -> [w1265]
          tunnel: w968 -> [w1260]
          tunnel: [w1259] -> w997
          shift-right: [w1256] -> _
          shift-left: 0.0 -> [w1257]
          i -> [w1269]
          stop <- w1262 stop-if-true
          n310 = Equal?(x=w1269, y=0) -> (x = y?=w1258:bool)
          n311 = call "Bis zum nächsten Vielfachen warten15"("Count(mSec)"=u32 50) -> ()  [unwired: 1 out]
          n312 = call "BigBen-01-16.vi"("MethodenStartzeit"=w1257, "Methodenstart?"=w1258, "Programmstart?"=w1267, "Zykluslängen [s]"=w1265, "MethodenStartZyklusNummern"=w1260) -> ("MethodenStartzeit"=w1256:dbl, "ZyklusNummernGesamt"=w1259:i32[])  [unwired: 2 in]
          n313 = global read "GVMethodenwechsel.vi" "Methodenwechsel?"() -> (w1261:bool)
          n314 = global read "gvbooleschRT.vi" "global stop RT"() -> (w1266:bool)
          n315 = local read "veränderte Methode benutzen"() -> (w1264:bool)
          n316 = Or(x=w1261, y=w1266) -> (x .or. y?=w1263:bool)
          n317 = Or(x=w1264, y=w1263) -> (x .or. y?=w1262:bool)
        }
        n318 = Bundle(w988, w987, w986, w985, "LHHeizen?"=w939, "ZPktFPGABoolesch"=w938, "FPGABoolesch"=w937, "ZeitpktFPGAPID"=w936, "FPGAPID"=w935, "ZeitpktFPGAFixp"=w934, "SHSetpoints"=w933, "t_PreMach1"=w932, "T_PreMach1"=w931, "t_PreMach2"=w930, "T_PreMach2"=w929, "ZeitpunkteMPV"=w925, "SPMPV"=w924, "t_MainMach1"=w912, "T_MainMach1"=w911, "t_MainMach2"=w910, "T_MainMach2"=w909) -> (w984:T24)  [unwired: 1 in]
        n319 = Index Array(array=w991, index=w916) -> (element=w915:T20)
        n320 = while {
          tunnel: w1010 -> [w1282]
          shift-right: [w1273] -> _
          shift-left: w915 -> [w1281]
          tunnel: w916 -> [w1279]
          shift-right: [w1271] -> w1009
          shift-left: w991 -> [w1280]
          tunnel: [w1272] -> w914
          stop <- w1275 stop-if-true
          n321 = call "Bis zum nächsten Vielfachen warten8"("Count(mSec)"=u32 500) -> ()  [unwired: 1 out]
          n322 = global read "GVMethodenwechsel.vi" "Methodenwechsel?"() -> (w1277:bool)
          n323 = global read "gvbooleschRT.vi" "global stop RT"() -> (w1276:bool)
          n324 = case shown="True" "Methode verändern" {
            tunnel: w1282 -> [_ w1304]
            tunnel: w1281 -> [w1301 w1303]
            tunnel: [w1301 w1302] -> w1273
            frame False {
            }
            frame True {
              n325 = call "methodeändern-11-15.vi"("Methode"=w1303, "Namen"=w1304) -> ("Methode"=w1302:T25)  [unwired: 1 in]
              n326 = property on="Methode verändern" class="Bool (strict)"("Value"=FALSE ("Methode verändern")) -> ()  [unwired: 2 in, 2 out]
            }
          }
          n327 = Compound Arithmetic op=OR(w1277, w1276, "veränderte Methode benutzen") -> (w1275:bool)
          n328 = case shown="True" "Methode speichern" {
            tunnel: w1273 -> [_ w1298]
            tunnel: w1280 -> [w1291 w1300]
            tunnel: w1279 -> [_ w1299]
            tunnel: [w1291 w1293] -> w1271
            frame False {
            }
            frame True {
              n329 = Replace Array Subset(array=w1300, new element=w1298, index=w1299) -> (w1293:T13)
              n330 = property on="Methode speichern" class="Bool (strict)"("Value"=FALSE ("Methode speichern")) -> ()  [unwired: 2 in, 2 out]
              n331 = Open/Create/Replace File(file path (use dialog)=path "c:/methoden.per" ("Dateipfad (Dialog verwenden)"), operation (0:open)=T14."replace" ("Operation (0:Öffnen)")) -> (refnum out=w1295:refnum<file>)  [unwired: 4 in, 2 out]
              n332 = Write to Binary File(file (use dialog)=w1295, data=w1293) -> (refnum out=w1292:refnum<file>)  [unwired: 4 in, 2 out]
              n333 = Close File(refnum=w1292) -> ()  [unwired: 1 in, 2 out]
            }
          }
          n334 = case shown="False" "veränderte Methode benutzen" {
            tunnel: w1273 -> [_ w1288]
            tunnel: [w1285 w1288] -> w1272
            tunnel: w1271 -> [w1287 _]
            frame False {
              n335 = local read "Methode"() -> (w1286:i32)
              n336 = Index Array(array=w1287, index=w1286) -> (element=w1285:T20)
            }
            frame True {
              n337 = flat-sequence {
                frame #0 {
                  n338 = call "Warten"("Count(mSec)"=u32 1100) -> ()  [unwired: 1 out]
                }
                frame #1 {
                  n339 = property on="veränderte Methode benutzen" class="Bool (strict)"("Value"=FALSE ("Methode verändern")) -> ()  [unwired: 2 in, 2 out]
                }
              }
            }
          }
        }
        n340 = Bundle(w973, w973, w973, w973) -> (w974:cluster{dbl[], dbl[], dbl[], dbl[]})  [unwired: 1 in]
        n341 = Bundle("ZyklusNummern"=w967, "ZeilennummernDIOs"=w983, "ZwangsDIO?"=w971, "ZeilennummernHorst"=w982, "ZwangsHorst?"=w972, "ZeileFPGABoolesch"=w981, "ZwangsFPGABoolesch?"=w970, "ZeileFPGAPID"=w980, "ZeileFPGAFixp"=w979, "ZeilePreMach1"=w978, "ZeilePreMach2"=w977, "ZeilennummerMPV"=w960, "ZeileMainMach1"=w904, "ZeileMainMach2"=w903, "ZwangsMPV?"=w888) -> (w976:T26)  [unwired: 1 in]
        n342 = call "arrayDoppelMoppel-11-15.vi"("verdoppeln"=i32[] [0, 1], "Traps/MachsKoeff2"=w892, "Traps/MachsKoeff1"=w896, "Traps/MachsKoeff0"=w902) -> ("Traps/MachsKoeff2"=w905:dbl[], "Traps/MachsKoeff1"=w906:dbl[], "Traps/MachsKoeff0"=w907:dbl[])  [unwired: 5 in]
        n343 = while "ZyklusSteuerung" {
          tunnel: w1001 -> [w1249]
          tunnel: w1002 -> [w1239]
          shift-right: [w1248] -> _
          shift-left: w976 -> [w1242]
          tunnel: w984 -> [w1246]
          tunnel: w907 -> [w1245]
          tunnel: w906 -> [w1244]
          tunnel: w905 -> [w1243]
          tunnel: w890 -> [w1247]
          shift-right: [w1241] -> _
          shift-left: errorcluster {"status"=FALSE, "code"=0, "source"=""} ("error out") -> [w1240]
          stop <- w1251 stop-if-true
          n344 = local read "veränderte Methode benutzen"() -> (w1252:bool)
          n345 = call "Bis zum nächsten Vielfachen warten11"("Count(mSec)"=u32 100) -> ()  [unwired: 1 out]
          n346 = global read "GVMethodenwechsel.vi" "Methodenwechsel?"() -> (w1254:bool)
          n347 = global read "gvbooleschRT.vi" "global stop RT"() -> (w1253:bool)
          n348 = call "ZyklussteuerungGV-01-17.vi"("Traps/MachKoeff0"=w1245, "DIOsNummern"=w1249, "error in"=w1240, "Traps/MachKoeff1"=w1244, "ServosWarmHigh (us)KaltHigh(us)"="ServosWarmHigh (us)KaltHigh(us)", "Traps/MachKoeff2"=w1243, "Schieberegister"=w1242, "Zeitpunkte/Setpoints"=w1246, "FPGA VI Reference In"=w1239, "MachKoeffs"=w1247) -> ("Schieberegister"=w1248:T27, "error out"=w1241:errorcluster)  [unwired: 4 in]
          "Zyklus" <- w1241
          n349 = Compound Arithmetic op=OR(w1254, w1253, w1252) -> (w1251:bool)
        }
        n350 = while {
          shift-right: [w1197] -> _
          shift-left: w974 -> [w1204]
          shift-right: [w1196] -> _
          shift-left: w974 -> [w1203]
          shift-right: [w1194] -> _
          shift-left: T17 {"Zyklus1"=0, "Zeitachse1"=0, "dargestellte Größe 1"=0, "Zyklus2"=0, "Zeitachse2"=0, "dargestellte Größe 2"=0} ("AnzeigeEinstellungen") -> [w1202]
          tunnel: w957 -> [w1172]
          shift-right: [w1168] -> _
          shift-left: w966 -> [w1167]
          shift-right: [w1163] -> _
          shift-left: w964 -> [w1165]
          shift-right: [w1152] -> _
          shift-left: w964 -> [w1164]
          shift-right: ["Detektor"] -> _
          shift-left: 0 ("Detektor") -> [w1161]
          tunnel: w885 -> [w1150]
          stop <- w1208 stop-if-true
          w1173 = 0.0 ("X-Achse.Bereich:Minimum")
          n351 = call "Bis zum nächsten Vielfachen warten14"("Count(mSec)"=u32 1000) -> ()  [unwired: 1 out]
          n352 = global read "GVMWHorst.vi" "MWHorst"() -> (w1101:dbl[])
          "MWHorst" <- w1101
          n353 = case shown="0, Default" "Detektor" {
            tunnel: [w1218 w1230] -> w1163
            tunnel: w1172 -> [w1217 w1232]
            tunnel: "Detektor" -> [w1212 w1226]
            tunnel: [w1216 w1231] -> w1170
            tunnel: [w1215 w1229] -> w1168
            frame 0, Default {
              n354 = Increment(x=w1212) -> (x+1=w1213:i32)
              n355 = Increment(x=w1213) -> (x+1=w1211:i32)
              n356 = global read "GVChroms.vi" "ECD1Chrom"() -> (w1214:dbl[])
              n357 = global read "GVaktuelleTDMS.vi" "aktuelleTDMS-DateiECD1"() -> (w1215:refnum<k34>)
              n358 = Index Array(array=w1217, index=w1211) -> (element=w1216:dbl)
              n359 = Array Size(array=w1214) -> (size(s)=w1220:i32)
              n360 = for {
                N: w1220 -> [_]
                tunnel: [w1221] -> w1219 mode=indexing
                i -> [w1224]
                n361 = To Double Precision Float(number=w1224) -> (double precision float=w1223:dbl)
                n362 = Divide(x=w1223, y=10.0) -> (x/y=w1221:dbl)
              }
              n363 = Bundle(w1219, "ECD1Chrom"=w1214) -> (w1218:cluster{dbl[], "ECD1Chrom":dbl[]})  [unwired: 1 in]
            }
            frame 1 {
              n364 = Increment(x=w1226) -> (x+1=w1227:i32)
              n365 = Increment(x=w1227) -> (x+1=w1225:i32)
              n366 = global read "GVChroms.vi" "ECD2Chrom"() -> (w1228:dbl[])
              n367 = global read "GVaktuelleTDMS.vi" "aktuelleTDMS-DateiECD2"() -> (w1229:refnum<k34>)
              n368 = Index Array(array=w1232, index=w1225) -> (element=w1231:dbl)
              n369 = Array Size(array=w1228) -> (size(s)=w1234:i32)
              n370 = for {
                N: w1234 -> [_]
                tunnel: [w1235] -> w1233 mode=indexing
                i -> [w1238]
                n371 = To Double Precision Float(number=w1238) -> (double precision float=w1237:dbl)
                n372 = Divide(x=w1237, y=10.0) -> (x/y=w1235:dbl)
              }
              n373 = Bundle(w1233, "ECD2Chrom"=w1228) -> (w1230:cluster{dbl[], "ECD2Chrom":dbl[]})  [unwired: 1 in]
            }
          }
          n374 = Equal?(x="Detektor", y=w1161) -> (x = y?=w1160:bool)
          n375 = Subtract(x="HK1YMax", y="HK1YMin") -> (x-y=w1188:dbl)
          n376 = Subtract(x="HK2YMax", y="HK2YMin") -> (x-y=w1183:dbl)
          n377 = Subtract(x="DetYMax", y="DetYMin") -> (x-y=w1178:dbl)
          n378 = Unbundle(w1150) -> ("Modul1/AI sicherer Bereich"=w1143:dbl[][], "Modul2/AI sicherer Bereich"=w1128:dbl[][], "Modul3/AI sicherer Bereich"=w1119:dbl[][], "Traps/Machs sicherer Bereich"=w1110:dbl[][], w1102:dbl[][], "Metavariablen grüner Bereich"=w1093:dbl[][])
          n379 = Index Array(array=w1102, index (col) #1=0 ("disabled index (col)"), index (col) #2=1 ("index (col)")) -> (element #1=w1106:dbl[], element #2=w1105:dbl[])  [unwired: 2 in]
          n380 = Greater Or Equal?(x=w1101, y=w1106) -> (x >= y?=w1104:bool[])
          n381 = Less Or Equal?(x=w1101, y=w1105) -> (x <= y?=w1103:bool[])
          n382 = And(x=w1104, y=w1103) -> (x .and. y?=→"HorstOK?":bool[])
          n383 = global read "GVMethodenwechsel.vi" "Methodenwechsel?"() -> (w1206:bool)
          n384 = global read "GVZeitenZyklen.vi" "ZyklusNummern"() -> (w1175:i32[])
          "ZyklusNummern" <- w1175
          n385 = global read "GVMetavariablen.vi" "Metavariablen"() -> (w1092:dbl[])
          "Metavariablen" <- w1092
          n386 = global read "gvbooleschRT.vi" "global stop RT"() -> (w1207:bool)
          n387 = global read "GVVentilposition.vi" "Ventilposition"() -> (→"Ventilposition":i32)
          n388 = Index Array(array=w1143, index (col) #1=0 ("disabled index (col)"), index (col) #2=1 ("index (col)")) -> (element #1=w1140:dbl[], element #2=w1138:dbl[])  [unwired: 2 in]
          n389 = Index Array(array=w1119, index (col) #1=0 ("disabled index (col)"), index (col) #2=1 ("index (col)")) -> (element #1=w1123:dbl[], element #2=w1122:dbl[])  [unwired: 2 in]
          n390 = Divide(x=w1188, y=10.0) -> (x/y=w1186:dbl)
          n391 = Divide(x=w1183, y=10.0) -> (x/y=w1181:dbl)
          n392 = Divide(x=w1178, y=20.0) -> (x/y=w1176:dbl)
          n393 = Index Array(array=w1128, index (col) #1=0 ("disabled index (col)"), index (col) #2=1 ("index (col)")) -> (element #1=w1132:dbl[], element #2=w1131:dbl[])  [unwired: 2 in]
          n394 = global read "GVZeitenZyklen.vi" "ZyklusNummernGesamt"() -> (→"ZyklusNummernGesamt":i32[])
          n395 = local read "veränderte Methode benutzen"() -> (w1205:bool)
          n396 = Or(x=w1206, y=w1207) -> (x .or. y?=w1209:bool)
          n397 = Index Array(array=w1093, index (col) #1=0 ("disabled index (col)"), index (col) #2=1 ("index (col)")) -> (element #1=w1097:dbl[], element #2=w1096:dbl[])  [unwired: 2 in]
          n398 = Greater Or Equal?(x=w1092, y=w1097) -> (x >= y?=w1095:bool[])
          n399 = Less Or Equal?(x=w1092, y=w1096) -> (x <= y?=w1094:bool[])
          n400 = global read "GVZeitenZyklen.vi" "Big Ben, Methodenzeit, Zykluszeit0, Zykluszeit1, Zykluszeit2A, Zykluszeit2B"() -> (w1155:dbl[])
          n401 = Or(x=w1209, y=w1205) -> (x .or. y?=w1208:bool)
          n402 = And(x=w1095, y=w1094) -> (x .and. y?=→"MVOK?":bool[])
          n403 = Index Array(array=w1110, index (col) #1=0 ("disabled index (col)"), index (col) #2=1 ("index (col)")) -> (element #1=w1114:dbl[], element #2=w1113:dbl[])  [unwired: 2 in]
          n404 = global read "GVHK1Hz.vi" "Mod1Mod2Mod3/AITrapsMachs1Hz"() -> (w1088:dbl[])
          n405 = Array Subset(array=w1088, index=0 ("Index"), length=32 ("Länge")) -> (w1139:dbl[])
          "AIs1" <- w1139
          n406 = Greater Or Equal?(x=w1139, y=w1140) -> (x >= y?=w1137:bool[])
          n407 = Less Or Equal?(x=w1139, y=w1138) -> (x <= y?=w1136:bool[])
          n408 = And(x=w1137, y=w1136) -> (x .and. y?=→"AIs1OK?":bool[])
          n409 = Array Subset(array=w1088, index=32 ("Index"), length=32 ("Länge")) -> (w1127:dbl[])
          "AIs2" <- w1127
          n410 = Greater Or Equal?(x=w1127, y=w1132) -> (x >= y?=w1130:bool[])
          n411 = Less Or Equal?(x=w1127, y=w1131) -> (x <= y?=w1129:bool[])
          n412 = And(x=w1130, y=w1129) -> (x .and. y?=→"AIs2OK?":bool[])
          n413 = Array Subset(array=w1088, index=64 ("Index"), length=32 ("Länge")) -> (w1118:dbl[])
          "AIs3" <- w1118
          n414 = Greater Or Equal?(x=w1118, y=w1123) -> (x >= y?=w1121:bool[])
          n415 = Less Or Equal?(x=w1118, y=w1122) -> (x <= y?=w1120:bool[])
          n416 = And(x=w1121, y=w1120) -> (x .and. y?=→"AIs3OK?":bool[])
          n417 = Array Subset(array=w1088, index=96 ("Index"), length=6 ("Länge")) -> (w1087:dbl[])
          "schnelle Heizungen" <- w1087
          n418 = Greater Or Equal?(x=w1087, y=w1114) -> (x >= y?=w1112:bool[])
          n419 = Less Or Equal?(x=w1087, y=w1113) -> (x <= y?=w1111:bool[])
          n420 = And(x=w1112, y=w1111) -> (x .and. y?=→"SHOK?":bool[])
          n421 = To Long Integer(number=w1155) -> (32bit integer=→"Big Ben, Methodenzeit, Zykluszeit0, Zykluszeit1, Zykluszeit2A, Zykluszeit2B":i32[])
          n422 = Equal?(x=w1168, y=w1167) -> (x = y?=w1166:bool)
          n423 = call "AnzeigeGV.vi"("veränderte Methode benutzen"=w1205, "Zykluslängen [s]"=w1172, "Cluster1"=w1204, "Big Ben, Methodenzeit, Zykluszeit0, Zykluszeit1, Zykluszeit2A, Zykluszeit2B"=w1155, "Zyklusnummern 0, 1, 2A, 2B"=w1175, "Cluster2"=w1203, "AnzeigeEinstellungen"=w1202, "dargestellte Größe 1"="dargestellte Größe 1", "Zeitachse1"="Zeitachse1", "dargestellte Größe 2"="dargestellte Größe 2", "Zeitachse2"="Zeitachse2") -> ("Anzeige2"=→"Housekeeping2":cluster{dbl[], dbl[]}, "Cluster1"=w1197:cluster{dbl[], dbl[], dbl[], dbl[]}, "x1Inkr"=w1192:dbl, "Cluster2"=w1196:cluster{dbl[], dbl[], dbl[], dbl[]}, "Anzeige1"=→"Housekeeping1":cluster{dbl[], dbl[]}, "AnzeigeEinstellungen"=w1194:T17, "x2Max"=w1156:dbl, "x2Inkr"=w1191:dbl, "x1Max"=w1157:dbl)  [unwired: 8 in]
          n424 = Divide(x=w1170, y=20.0) -> (x/y=w1171:dbl)
          n425 = Select(t=w1164, s=w1166, f=w1165) -> (s? t:f=w1159:cluster{dbl[], dbl[]})
          n426 = property on="Housekeeping1" class="XYGraph (strict)"("XScale.Minimum"=w1173, "XScale.Maximum"=w1157, "XScale.Increment"=w1192, "YScale.Minimum"="HK1YMin", "YScale.Maximum"="HK1YMax", "YScale.Increment"=w1186) -> ()  [unwired: 2 in, 2 out]
          n427 = property on="Housekeeping2" class="XYGraph (strict)"("XScale.Minimum"=w1173, "XScale.Maximum"=w1156, "XScale.Increment"=w1191, "YScale.Minimum"="HK2YMin", "YScale.Maximum"="HK2YMax", "YScale.Increment"=w1181) -> ()  [unwired: 2 in, 2 out]
          n428 = property on="Detektor 2" class="XYGraph (strict)"("XScale.Minimum"=w1173, "XScale.Maximum"=w1170, "XScale.Increment"=w1171, "YScale.Minimum"="DetYMin", "YScale.Maximum"="DetYMax", "YScale.Increment"=w1176) -> ()  [unwired: 2 in, 2 out]
          n429 = Select(t=w1159, s=w1160, f=cluster{dbl[], dbl[]} {[], []} ("s? t:f")) -> (s? t:f=w1152:cluster{dbl[], dbl[]})
          n430 = Build Array(w1163, w1152) -> (→"Detektor 2":cluster{dbl[], "ECD2Chrom":dbl[]}[])
        }
        n431 = global read "GVZeitenZyklen.vi" "Big Ben, Methodenzeit, Zykluszeit0, Zykluszeit1, Zykluszeit2A, Zykluszeit2B"() -> (w963:dbl[])
        n432 = Index Array(array=w963, index=3 ("Index")) -> (element=w961:dbl)
        n433 = while {
          tunnel: w1005 -> [w1032]
          tunnel: w1004 -> [w1031]
          tunnel: w926 -> [w1046]
          shift-right: [w1047] -> w998
          shift-left: w1003 -> [w1048]
          tunnel: w923 -> [w1042]
          tunnel: w922 -> [w1036]
          shift-right: [w1033] -> _
          shift-left: w961 -> [w1037]
          stop <- w1049 stop-if-true
          n434 = Less?(x=w1037, y=w1042) -> (x < y?=w1040:bool)
          n435 = Less?(x=w1037, y=w1036) -> (x < y?=w1038:bool)
          n436 = call "Bis zum nächsten Vielfachen warten13"("Count(mSec)"=u32 100 ("Zu wartende ms")) -> ()  [unwired: 1 out]
          n437 = global read "GVMethodenwechsel.vi" "Methodenwechsel?"() -> (w1051:bool)
          n438 = global read "gvbooleschRT.vi" "global stop RT"() -> (w1052:bool)
          n439 = local read "veränderte Methode benutzen"() -> (w1050:bool)
          n440 = global read "GVZeitenZyklen.vi" "Big Ben, Methodenzeit, Zykluszeit0, Zykluszeit1, Zykluszeit2A, Zykluszeit2B"() -> (w1044:dbl[])
          n441 = Compound Arithmetic op=OR(w1052, w1051, w1050) -> (w1049:bool)
          n442 = Index Array(array=w1044, index=3 ("Index")) -> (element=w1033:dbl)
          n443 = Greater Or Equal?(x=w1033, y=w1042) -> (x >= y?=w1041:bool)
          n444 = Greater Or Equal?(x=w1033, y=w1036) -> (x >= y?=w1039:bool)
          n445 = And(x=w1039, y=w1038) -> (x .and. y?=w1035:bool)
          n446 = And(x=w1041, y=w1040) -> (x .and. y?=w1030:bool)
          n447 = Or(x=w1030, y=w1035) -> (x .or. y?=w1034:bool)
          n448 = And(x=w1046, y=w1034) -> (x .and. y?=w1045:bool)
          n449 = case shown="True" w1045 {
            tunnel: w1048 -> [w1054 w1055]
            tunnel: [w1054 w1059] -> w1047
            tunnel: w1032 -> [_ w1058]
            tunnel: w1031 -> [_ w1057]
            tunnel: w1030 -> [_ w1056]
            frame False {
            }
            frame True {
              n450 = call "MSDateienSchicken12-15.vi"("MSNummer"=w1055, "MSa?"=w1056, "Dateipfad:fromcriordy"=w1057, "Dateipfad:fromcriocmd"=w1058) -> ()  [unwired: 1 in]
              n451 = Increment(x=w1055) -> (x+1=w1059:i32)
            }
          }
        }
      }
      n452 = Add Array Elements(numeric array=w477) -> (sum=w487:i32)
      n453 = Index Array(array=w477, index #1=0 ("Index"), index #2=1 ("Index")) -> (element #1=w498:i32, element #2=w496:i32)
      n454 = Split 1D Array(array=w476, index=w498) -> (first subarray=w502:dbl[], second subarray=w506:dbl[])
      n455 = Split 1D Array(array=w474, index=w498) -> (first subarray=w505:string[], second subarray=w507:string[])
      n456 = Split 1D Array(array=w475, index=w498) -> (first subarray=w495:string[], second subarray=w497:string[])
      n457 = Initialize Array(-1.0 ("Element"), w487) -> (w472:dbl[])
      n458 = Split 1D Array(array=w507, index=w496) -> (first subarray=w504:string[], second subarray=w503:string[])
      n459 = Split 1D Array(array=w506, index=w496) -> (first subarray=w501:dbl[], second subarray=w500:dbl[])
      n460 = Split 1D Array(array=w497, index=w496) -> (first subarray=w494:string[], second subarray=w493:string[])
      n461 = Bundle(w505, w504, w503, w502, w501, w500) -> (w499:T28)  [unwired: 1 in]
      n462 = Bundle(w495, w494, w493) -> (w492:cluster{string[], string[], string[]})  [unwired: 1 in]
      n463 = Initialize Array(0.0, 8 ("Dimension")) -> (w422:dbl[])
      n464 = Bundle(w491, w491, w491) -> (w490:cluster{i32, i32, i32})  [unwired: 1 in]
      n465 = Initialize Array("x", 8 ("Dimension")) -> (w427:string[])
      n466 = case shown="True" TRUE ("SerielleKomm.") {
        tunnel: bool[] [TRUE, TRUE, TRUE, TRUE, TRUE, TRUE, TRUE, TRUE] -> [_ w564]
        tunnel: w427 -> [_ w563]
        tunnel: w499 -> [_ w562]
        tunnel: w498 -> [_ w561]
        tunnel: w496 -> [_ w560]
        tunnel: w492 -> [_ w559]
        tunnel: w490 -> [_ w558]
        tunnel: w489 -> [_ w557]
        tunnel: w476 -> [_ w556]
        tunnel: w473 -> [_ w555]
        tunnel: w472 -> [_ w554]
        tunnel: w471 -> [_ w551]
        tunnel: w450 -> [_ w553]
        tunnel: w422 -> [_ w552]
        tunnel: w421 -> [_ w550]
        frame False {
        }
        frame True {
          n467 = while {
            tunnel: w551 -> [w575]
            tunnel: w550 -> [w568]
            shift-right: [w567] -> _
            shift-left: errorcluster {"status"=FALSE, "code"=0, "source"=""} ("error out") -> [w566]
            stop <- w577 stop-if-true
            n468 = String To Byte Array(string=w568) -> (unsigned byte array=w571:u8[])
            n469 = call "Warten6"("Count(mSec)"=u32 500) -> ()  [unwired: 1 out]
            n470 = Join Numbers(hi=w571, lo=u8 5) -> ((hi.lo)=w573:u16[])
            n471 = Join Numbers(hi=w571, lo=u8 6) -> ((hi.lo)=w569:u16[])
            n472 = xnode "Invoke Method"("FPGA VI Reference In"=w575, "error in"=w566, "Data"=w573) -> ("FPGA VI Reference Out"=w572:refnum<k20>, "error out"=w565:errorcluster)  [unwired: 1 in, 1 out]
            n473 = xnode "Invoke Method"("FPGA VI Reference In"=w572, "error in"=w565, "Data"=w569) -> ("error out"=w567:errorcluster)  [unwired: 1 in, 2 out]
            "FIFOwriteRS485" <- w567
            n474 = global read "gvbooleschRT.vi" "global stop RT"() -> (w577:bool)
          }
          n475 = while {
            shift-right: [w715] -> _
            shift-left: w564 -> [w730]
            shift-right: [w734] -> _
            shift-left: w554 -> [w740]
            tunnel: w551 -> [w729]
            shift-right: [w716] -> _
            shift-left: w563 -> [w718]
            tunnel: w555 -> [w720]
            tunnel: w556 -> [w717]
            shift-right: [w721] -> _
            shift-left: w557 -> [w736]
            tunnel: w561 -> [w738]
            tunnel: w560 -> [w739]
            tunnel: w562 -> [w741]
            tunnel: w559 -> [w723]
            shift-right: [w722] -> _
            shift-left: w558 -> [w724]
            shift-right: [w727] -> _
            shift-left: w553 -> [w728]
            shift-right: [w731] -> _
            shift-left: w552 -> [w732]
            shift-right: [w712] -> _
            shift-left: errorcluster {"status"=FALSE, "code"=0, "source"=""} ("error out") -> [w711]
            stop <- w735 stop-if-true
            n476 = for {
              tunnel: w730 -> [w745] mode=indexing
              tunnel: w732 -> [w742] mode=indexing
              tunnel: [w749] -> w731 mode=indexing
              tunnel: [w746] -> w725 mode=indexing
              n477 = global read "GVZeitenZyklen.vi" "Big Ben, Methodenzeit, Zykluszeit0, Zykluszeit1, Zykluszeit2A, Zykluszeit2B"() -> (w752:dbl[])
              n478 = Index Array(array=w752, index=0 ("Index")) -> (element=w750:dbl)
              n479 = Subtract(x=w750, y=w742) -> (x-y=w748:dbl)
              n480 = Greater?(x=w748, y=0.1) -> (0:w744:bool)
              n481 = Or(x=w745, y=w744) -> (x .or. y?=w743:bool)
              n482 = Select(t=w744, s=w744, f=w745) -> (s? t:f=w746:bool)
              n483 = Select(t=w750, s=w743, f=w742) -> (s? t:f=w749:dbl)
            }
            n484 = global read "GVHorstSP.vi" "HorstSP"() -> (w734:dbl[])
            n485 = Not Equal?(x=w734, y=w740) -> (x != y?=w737:bool)
            n486 = call "NeueSP.vi"("Anzahl2"=w739, "Anzahl1"=w738, "AlteSP"=w740, 7:"NeueSP"=w734, "BefehleCluster"=w736, 10:"NeueSP"=w737, "ClusterFest"=w741) -> ("BefehleCluster"=w726:T29)  [unwired: 4 in]
            n487 = call "Warten3"("Count(mSec)"=u32 50) -> ()  [unwired: 1 out]
            n488 = call "MPVSenden-01-17.vi"("Ventilposition"=w728, "error in"=w711, "FPGA VI Reference In"=w729) -> ("Ventilposition"=w727:i32, "error out"=w714:errorcluster, "FPGA VI Reference Out"=w710:refnum<k20>)
            n489 = call "Senden-01-17.vi"("error in"=w714, "BefehlsCluster"=w726, "AbfragenCluster"=w723, "Abfragenr.Cluster"=w724, "Senden?"=w725, "FPGA VI Reference In"=w710) -> ("BefehlsCluster"=w721:T29, "error out"=w713:errorcluster, "Senden?"=w719:bool[], "Abfragenr.Cluster"=w722:cluster{i32, i32, i32})  [unwired: 1 in]
            n490 = call "SeriellRead-01-17.vi"("SkalierungsfaktorHorst"=w717, "VorwortHorst"=w720, "error in"=w713, "Zwischenspeicher"=w718, "Senden?"=w719, "FPGA VI Reference In"=w710) -> ("Senden?"=w715:bool[], "Zwischenspeicher"=w716:string[], "error out"=w712:errorcluster)  [unwired: 3 in]
            "SerielleKomm." <- w712
            n491 = global read "gvbooleschRT.vi" "global stop RT"() -> (w735:bool)
          }
        }
      }
      n492 = flat-sequence {
        frame #0 {
          n493 = global write "Emulate Licor output GV.vi" "Emulator an?"(FALSE ("Emulator an?")) -> ()
        }
        frame #1 {
          n494 = control-ref of="GUI_Cluster_Parameter"() -> (w520:refnum<vi>)
          n495 = control-ref of="GUI_Cluster_Graph"() -> (w521:refnum<vi>)
          n496 = control-ref of="GUI_Cluster_sdv"() -> (w519:refnum<vi>)
          n497 = call "licore (main).vi"("GUI_Cluster_Graph (extern)"=w521, "GUI_Cluster_Parameter (extern)"=w520, "GUI_Cluster_sdv (extern)"=w519) -> ()  [unwired: 13 in]
        }
      }
    }
    frame #2 {
      n498 = xnode "Read/Write Control"("FPGA VI Reference In"=w1335, "global stop"=TRUE) -> ("FPGA VI Reference Out"=w1334:refnum<k20>)  [unwired: 1 in, 1 out]
      n499 = xnode "Close FPGA VI Reference"("FPGA VI Reference In"=w1334) -> ()  [unwired: 1 in, 1 out]
    }
    frame #3 {
    }
    frame #4 {
    }
  }
